vi "Farming Robot V4.vi"() -> ()   [LabVIEW 2021]
uses:
  <vilib>/myRIO/Instrument Drivers/Onboard IO/DIO/typedefs/DIO Reference.ctl
  <vilib>/myRIO/Common/Instrument Driver Framework/Utilities/typedefs/myRIO Generic Hardware Reference.ctl
  <vilib>/myRIO/Common/Instrument Driver Framework/Utilities/typedefs/Hardware Version Enum.ctl
  <vilib>/myRIO/Common/Instrument Driver Framework/Utilities/typedefs/myRIO v1.0 Reference.ctl
  <vilib>/myRIO/Common/Instrument Driver Framework/Utilities/typedefs/Generic FPGA Reference.ctl
  <vilib>/myRIO/Common/Instrument Driver Framework/myRIO v1.0/DIO/typedefs/DIO Channels List.ctl
  <vilib>/myRIO/Common/Instrument Driver Framework/myRIO v1.0/DIO/typedefs/DIO Channels Enum.ctl
  <vilib>/userDefined/High Color/nirio_resource_hc.ctl
  <vilib>/myRIO/Instrument Drivers/Onboard IO/PWM/typedefs/PWM Reference.ctl
  <vilib>/myRIO/Common/Instrument Driver Framework/myRIO v1.0/PWM/typedefs/PWM Channels Enum.ctl
  <vilib>/myRIO/Instrument Drivers/Onboard IO/PWM/typedefs/PWM Configuration.ctl
  <vilib>/myRIO/Instrument Drivers/Onboard Devices/Accelerometer/typedefs/Accelerometer Reference.ctl
  <vilib>/myRIO/Common/Instrument Driver Framework/myRIO v1.0/Accelerometer/typedefs/Accelerometer Channels List.ctl
  <vilib>/myRIO/Common/Instrument Driver Framework/myRIO v1.0/Accelerometer/typedefs/Accelerometer Channels Enum.ctl
  <vilib>/myRIO/Common/Instrument Driver Framework/Utilities/vis/Is FPGA Ref Available.vi
  <vilib>/myRIO/Common/Instrument Driver Framework/myRIO v1.0/DIO/vis/myRIO v1.1 Open DIO.vi
  <vilib>/myRIO/Instrument Drivers/Onboard IO/DIO/vis/Write.vi
  <vilib>/myRIO/Common/Instrument Driver Framework/myRIO v1.0/Accelerometer/vis/myRIO v1.1 Open Accelerometer.vi
  <vilib>/myRIO/Instrument Drivers/Onboard Devices/Accelerometer/vis/Read.vi
  <vilib>/myRIO/Common/Instrument Driver Framework/myRIO v1.0/PWM/vis/myRIO v1.1 Open PWM.vi
  <vilib>/myRIO/Instrument Drivers/Onboard IO/PWM/vis/Set Duty Cycle and Frequency.vi
  <vilib>/myRIO/Common/Instrument Driver Framework/Utilities/vis/Validate Channels.vi
  <vilib>/myRIO/Common/Instrument Driver Framework/myRIO v1.0/DIO/vis/myRIO v1.0 Reserve DIO.vi
  <vilib>/myRIO/Common/Instrument Driver Framework/myRIO v1.0/Accelerometer/vis/myRIO v1.0 Reserve Accelerometer.vi
  <vilib>/myRIO/Common/Instrument Driver Framework/myRIO v1.0/PWM/vis/myRIO v1.0 Reserve PWM.vi
  <vilib>/myRIO/Common/Instrument Driver Framework/myRIO v1.0/Resource Manager/vis/myRIO v1.0 Reserve Channel List.vi
  <vilib>/myRIO/Common/Instrument Driver Framework/myRIO v1.0/DIO/vis/myRIO v1.0 Build MUX Configuration DIO.vi
  <vilib>/myRIO/Common/Instrument Driver Framework/myRIO v1.0/Accelerometer/vis/myRIO v1.0 Build MUX Configuration Accelerometer.vi
  <vilib>/myRIO/Common/Instrument Driver Framework/myRIO v1.0/PWM/vis/myRIO v1.0 Build MUX Configuration PWM.vi
  <vilib>/myRIO/Common/Instrument Driver Framework/myRIO v1.0/Resource Manager/vis/myRIO v1.0 Reserve Channel.vi
  <vilib>/myRIO/Common/Instrument Driver Framework/myRIO v1.0/Resource Manager/vis/myRIO v1.0 Unreserve Channel.vi
  <vilib>/myRIO/Common/Instrument Driver Framework/myRIO v1.0/Resource Manager/vis/myRIO v1.0 Create Configuration List.vi
  <vilib>/myRIO/Common/Instrument Driver Framework/myRIO v1.0/Resource Manager/vis/myRIO v1.0 Build Mutex Name.vi
  <vilib>/Utility/VariantDataType/GetNumericInfo.vi
  <vilib>/Utility/error.llb/Error Cluster From Error Code.vi
  <vilib>/myRIO/Common/Instrument Driver Framework/myRIO v1.0/myRIO v1.1 Open.vi
  <vilib>/myRIO/Common/Instrument Driver Framework/Utilities/vis/IO Manager.vi
  <vilib>/myRIO/Common/Instrument Driver Framework/Utilities/vis/Configuration Manager.vi
  <vilib>/myRIO/Common/Instrument Driver Framework/myRIO v1.0/Resource Manager/vis/myRIO v1.0 Configure IO.vi
  <vilib>/myRIO/Common/Instrument Driver Framework/myRIO v1.0/myRIO v1.0 Close.vi
  <vilib>/myRIO/Common/Instrument Driver Framework/myRIO v1.0/DIO/vis/myRIO v1.0 Write DIO.vi
  <vilib>/myRIO/Common/Instrument Driver Framework/myRIO v1.0/PWM/vis/myRIO v1.0 Write PWM.vi
  <vilib>/myRIO/Common/Instrument Driver Framework/myRIO v1.0/Accelerometer/vis/myRIO v1.0 Get Scaling Constant Accelerometer.vi
  <vilib>/myRIO/Common/Instrument Driver Framework/myRIO v1.0/Accelerometer/vis/myRIO v1.0 Read Accelerometer.vi
  <vilib>/myRIO/Express VI/Onboard Devices/LED/LED Express VI.xnode
  <vilib>/myRIO/Instrument Drivers/Onboard IO/DIO/vis/myRIO DIO Open.xnode
  <vilib>/myRIO/Express VI/Onboard IO/DO/DO Express VI.xnode
  <vilib>/myRIO/Express VI/Onboard IO/PWM/PWM Express VI.xnode
  <vilib>/myRIO/Instrument Drivers/Onboard IO/PWM/vis/myRIO PWM Open.xnode
  <vilib>/myRIO/Express VI/Onboard Devices/Accelerometer/Accelerometer Express VI.xnode
  <vilib>/myRIO/Instrument Drivers/Onboard Devices/Accelerometer/vis/myRIO Accelerometer Open.xnode
  <vilib>/myRIO/Instrument Drivers/Onboard IO/DIO/DIO.lvlib
  <vilib>/myRIO/Instrument Drivers/Onboard IO/PWM/PWM.lvlib
  <vilib>/myRIO/Instrument Drivers/Onboard Devices/Accelerometer/Accelerometer.lvlib
  <vilib>/Analysis/NI_AALPro.lvlib
panel:
  out "States":T1(ring)
  out "pulse width 2":dbl
  out "Angle 2":dbl
  out "pulse width 1":dbl
  out "Angle 1":dbl
  in  "Start Farming":bool
  out "Watering":bool
  out "Seeding\nUp":bool
  out "Seeding\nDown":bool
  out "Switching\nMode":bool
  out "Drill Up":bool
  out "Drill Down":bool
  out "Intialize":bool
  out "Message":string
  in  "stop":bool
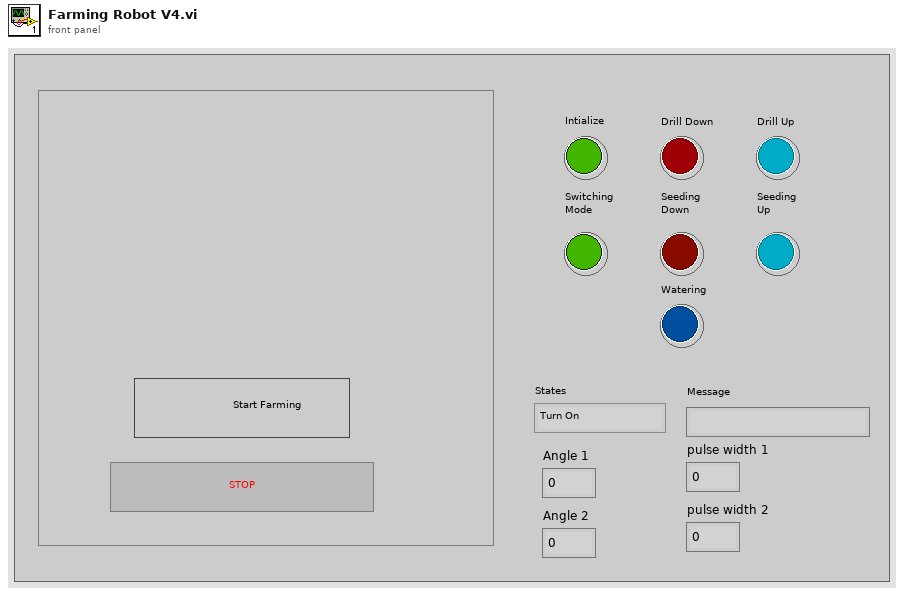
[diagram p1: front panel]
types:
  T1 = enum16{"Turn On", "IDLE", "Drive", "Down-Drilling", "Up-Drilling", "Switch-Seeding", "Down-Seeding", "Seeding", "Up-Seeding", "Switch-Watering", "Watering", "Filling", "Fell Off", "Stop"}
  T2 = typedef "DIO.lvlib/DIO Reference.ctl" = cluster{"myRIO Reference":T3, "DIO Channels List":T7}
  T3 = typedef "myRIO Generic Hardware Reference.ctl" = cluster{"myRIO Model":T4, "myRIO Hardware Reference":T5}
  T4 = typedef "Hardware Version Enum.ctl" = enum16{"Unknown", "myRIO-1900", "myRIO-1950", "roboRIO", "NI ELVIS RIO CM", "ELVIS III"}
  T5 = typedef "myRIO v1.0 Reference.ctl" = cluster{"Generic FPGA Reference":T6, "Allow multiple opens":bool}
  T6 = typedef "Generic FPGA Reference.ctl" = refnum<k20>
  T7 = typedef "DIO Channels List.ctl" = T8[]
  T8 = typedef "DIO Channels Enum.ctl" = enum16{"Not Connected", "C/DIO0", "C/DIO1", "C/DIO2", "C/DIO3", "C/DIO4", "C/DIO5", "C/DIO6", "C/DIO7", "A/DIO0", "A/DIO1", "A/DIO2", "A/DIO3", "A/DIO4", "A/DIO5", "A/DIO6", "A/DIO7", "A/DIO8", "A/DIO9", "A/DIO10", "A/DIO11", "A/DIO12", "A/DIO13", "A/DIO14", "A/DIO15", "A/DIO16", "A/DIO17", "A/DIO18", "A/DIO19", "B/DIO0", "B/DIO1", "B/DIO2", "B/DIO3", "B/DIO4", "B/DIO5", "B/DIO6", "B/DIO7", "B/DIO8", "B/DIO9", "B/DIO10", "B/DIO11", "B/DIO12", "B/DIO13", "B/DIO14", "B/DIO15", "B/DIO16", "B/DIO17", "B/DIO18", "B/DIO19", "LED0", "LED1", "LED2", "LED3", "Button0", "DIO/DIO0", "DIO/DIO1", "DIO/DIO2", "DIO/DIO3", "DIO/DIO4", "DIO/DIO5", "DIO/DIO6", "DIO/DIO7", "DIO/DIO8", "DIO/DIO9", "SPI/CS0", "SPI/CS1", "SPI/CS2", "SPI/CS3", "LED RADIO (Green)", "LED RADIO (Red)", "LED COMM (Green)", "LED COMM (Red)", "LED MODE (Green)", "LED MODE (Red)"}
  T9 = typedef "nirio_resource_hc.ctl" = tag
  T10 = typedef "Accelerometer.lvlib/Accelerometer Reference.ctl" = cluster{"myRIO Reference":T3, "Accelerometer Channels List":T11, "LSB Weight":dbl}
  T11 = typedef "Accelerometer Channels List.ctl" = T12[]
  T12 = typedef "Accelerometer Channels Enum.ctl" = enum16{"Not Connected", "X-Axis", "Y-Axis", "Z-Axis"}
  T13 = typedef "PWM.lvlib/PWM Reference.ctl" = cluster{"myRIO Reference":T3, "PWM Channels Enum":T14, "PWM Configuration":T15}
  T14 = typedef "PWM Channels Enum.ctl" = enum16{"Not Connected", "C/PWM0", "C/PWM1", "A/PWM0", "A/PWM1", "A/PWM2", "A/PWM3", "A/PWM4", "A/PWM5", "A/PWM6", "A/PWM7", "A/PWM8", "A/PWM9", "A/PWM10", "A/PWM11", "A/PWM12", "A/PWM13", "A/PWM14", "A/PWM15", "A/PWM16", "A/PWM17", "A/PWM18", "A/PWM19", "B/PWM0", "B/PWM1", "B/PWM2", "B/PWM3", "B/PWM4", "B/PWM5", "B/PWM6", "B/PWM7", "B/PWM8", "B/PWM9", "B/PWM10", "B/PWM11", "B/PWM12", "B/PWM13", "B/PWM14", "B/PWM15", "B/PWM16", "B/PWM17", "B/PWM18", "B/PWM19", "PWM/PWM0", "PWM/PWM1", "PWM/PWM2", "PWM/PWM3", "PWM/PWM4", "PWM/PWM5", "PWM/PWM6", "PWM/PWM7", "PWM/PWM8", "PWM/PWM9"}
  T15 = typedef "PWM.lvlib/PWM Configuration.ctl" = cluster{"Frequency":dbl, "Duty Cycle":dbl}
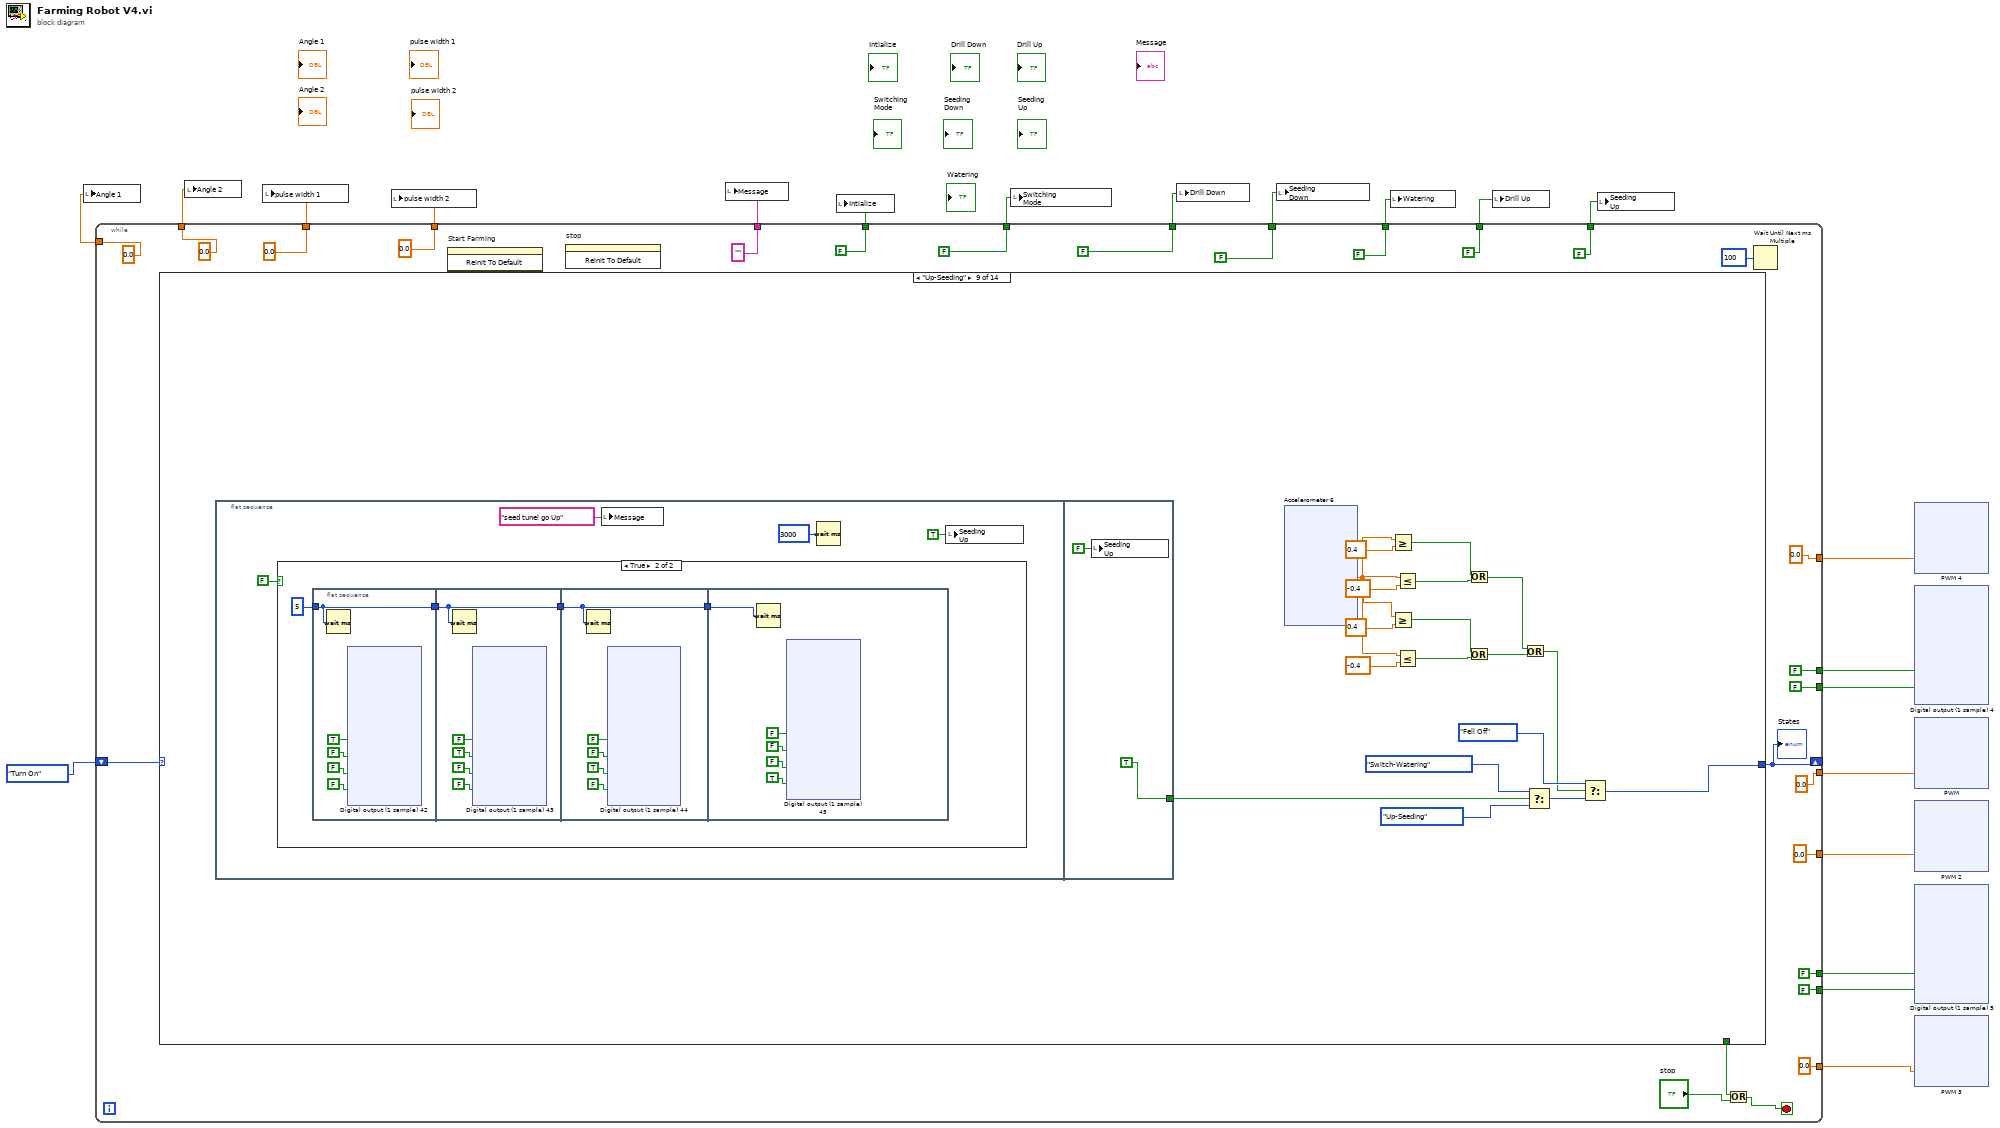
[diagram p0: block diagram]
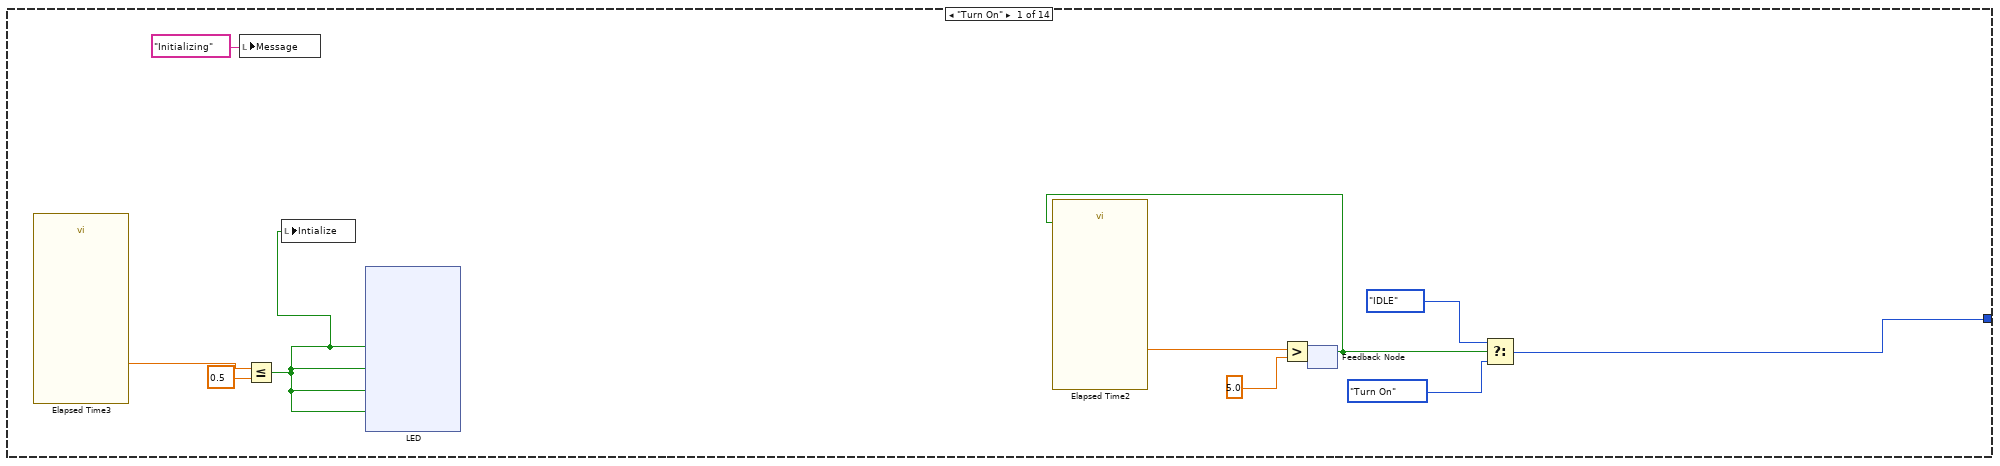
[diagram p2: hidden frame]
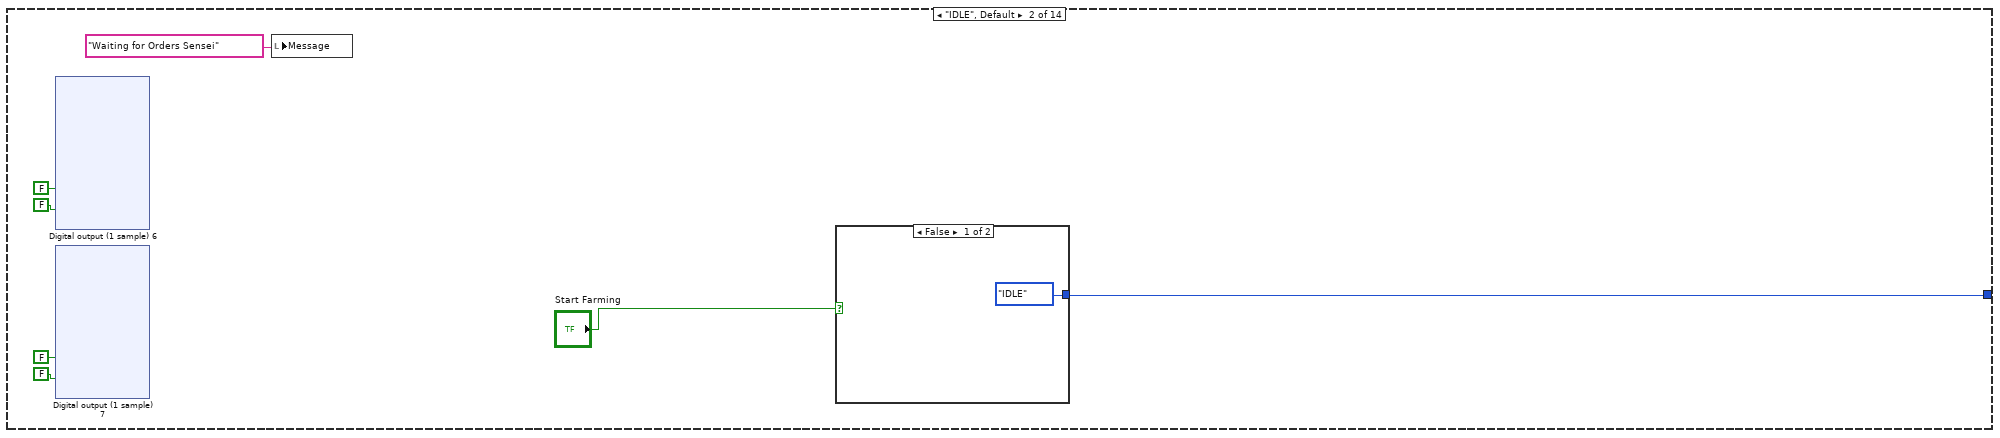
[diagram p3: hidden frame]
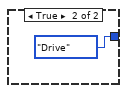
[diagram p4: hidden frame]
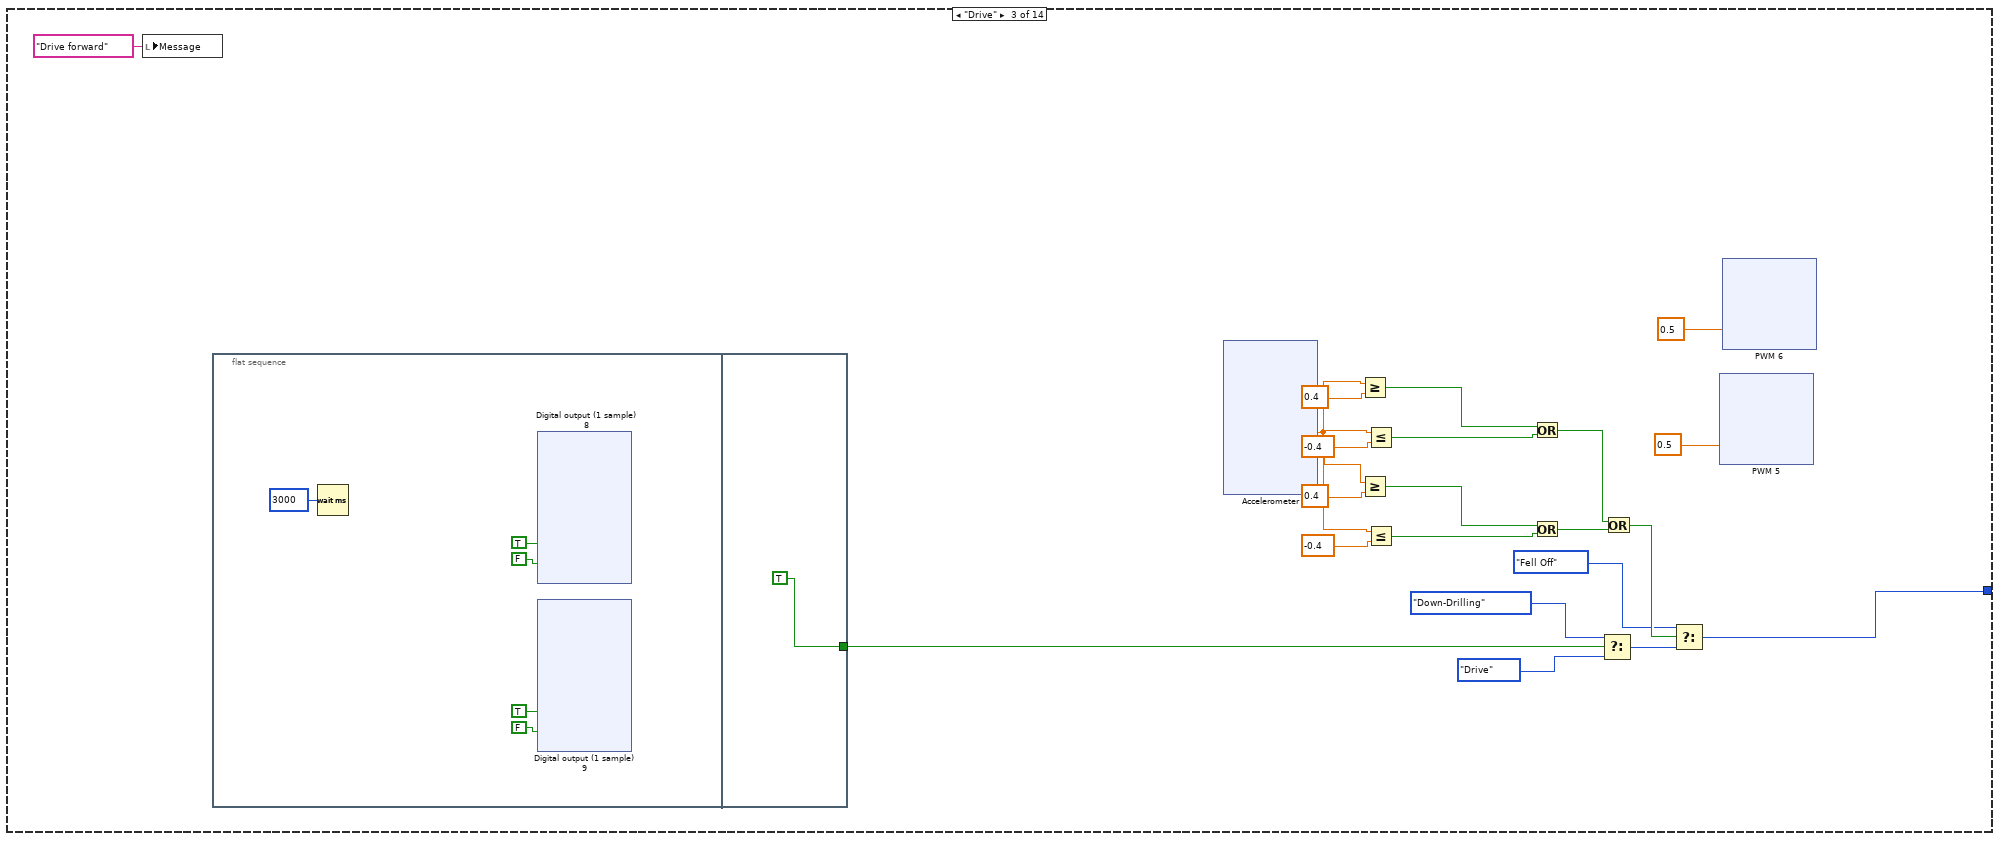
[diagram p5: hidden frame]
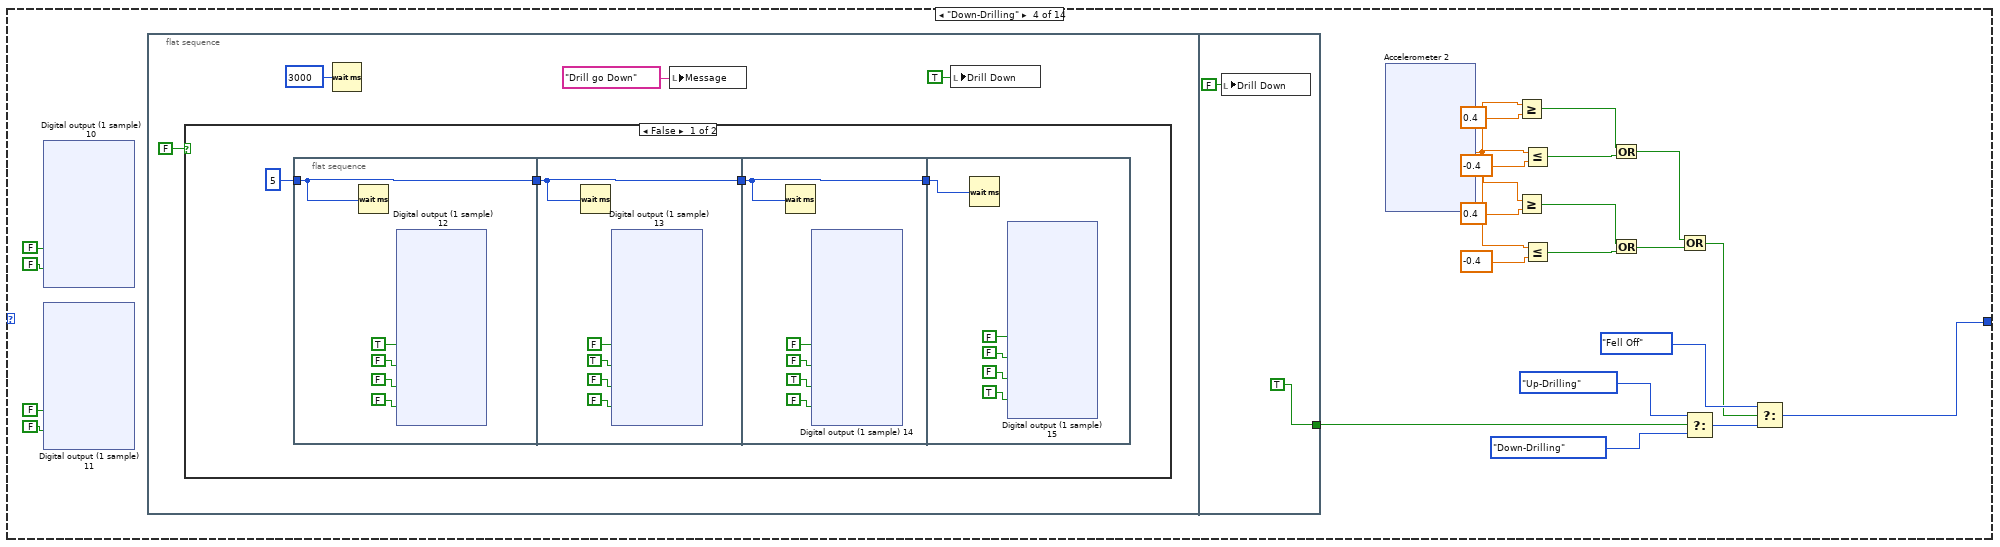
[diagram p6: hidden frame]
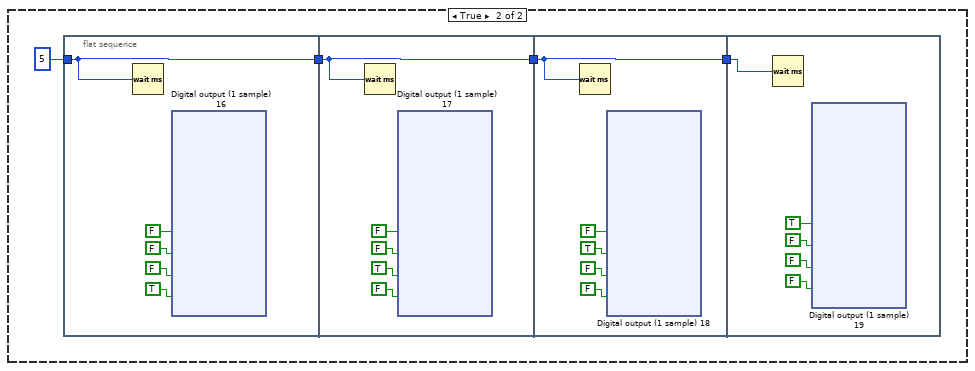
[diagram p7: hidden frame]
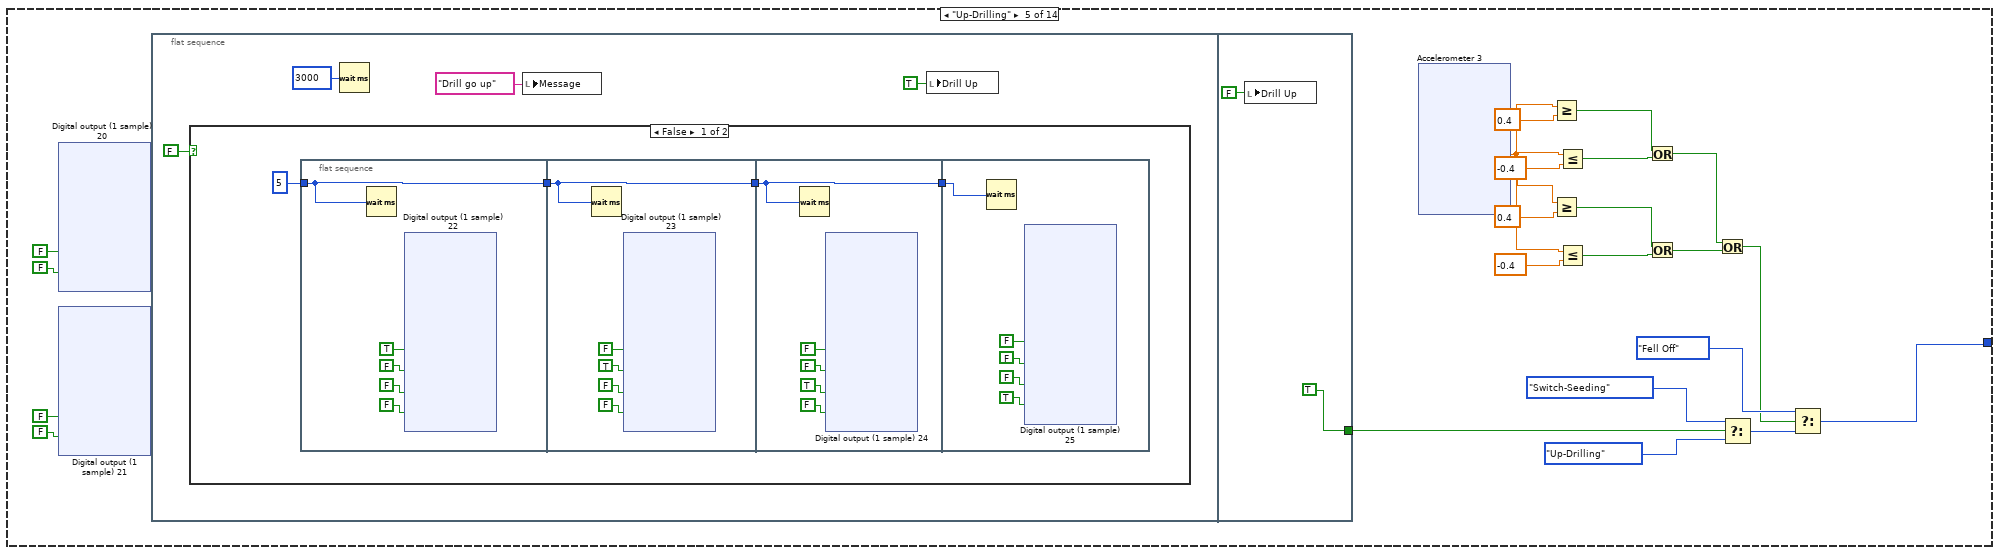
[diagram p8: hidden frame]
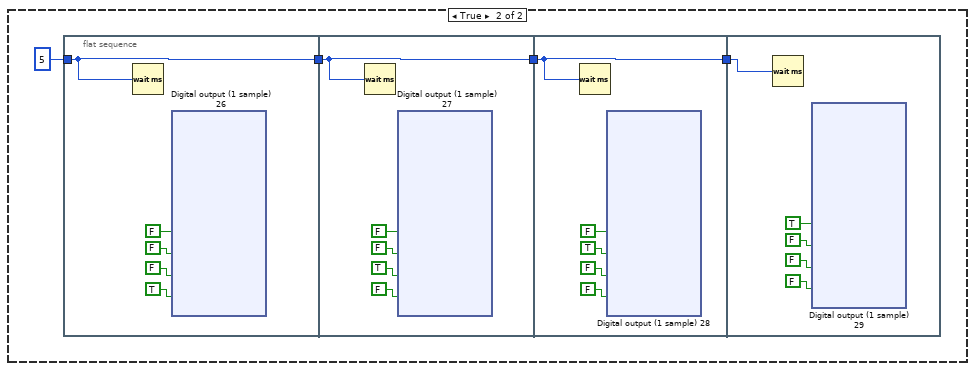
[diagram p9: hidden frame]
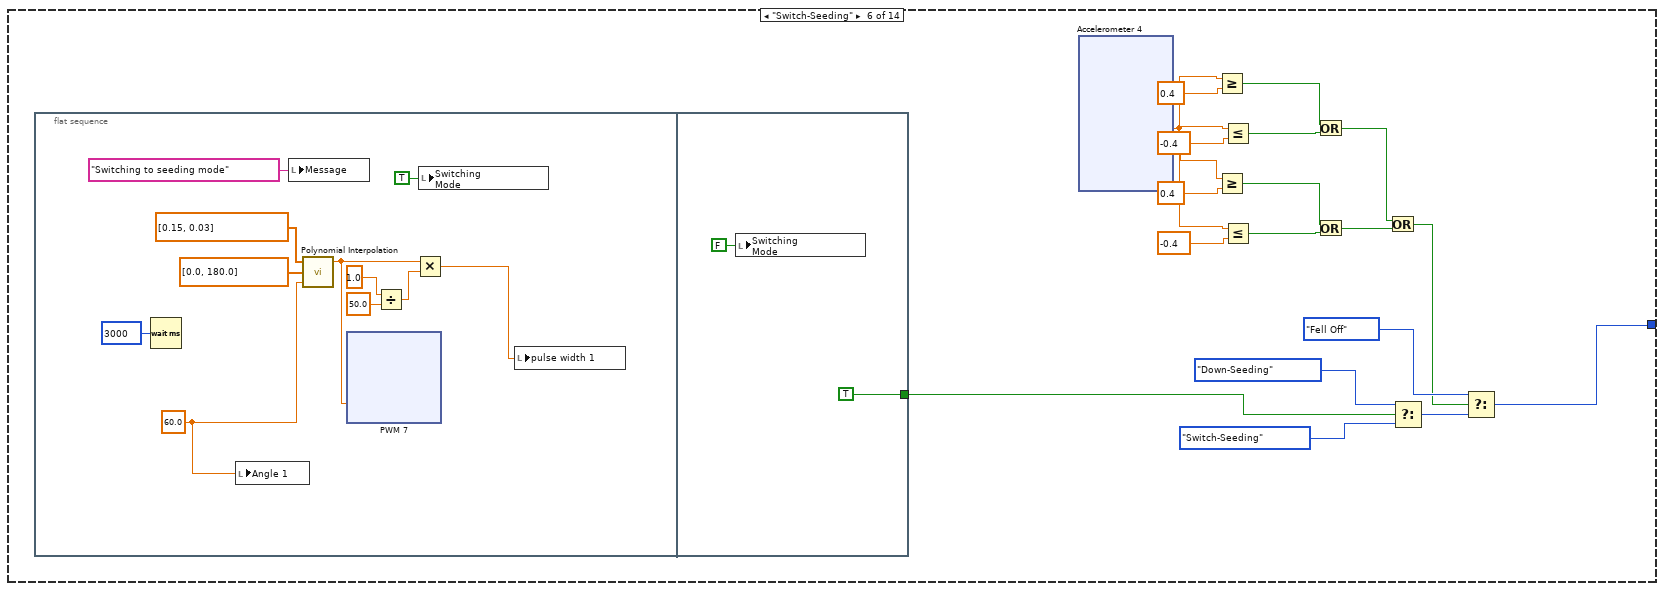
[diagram p10: hidden frame]
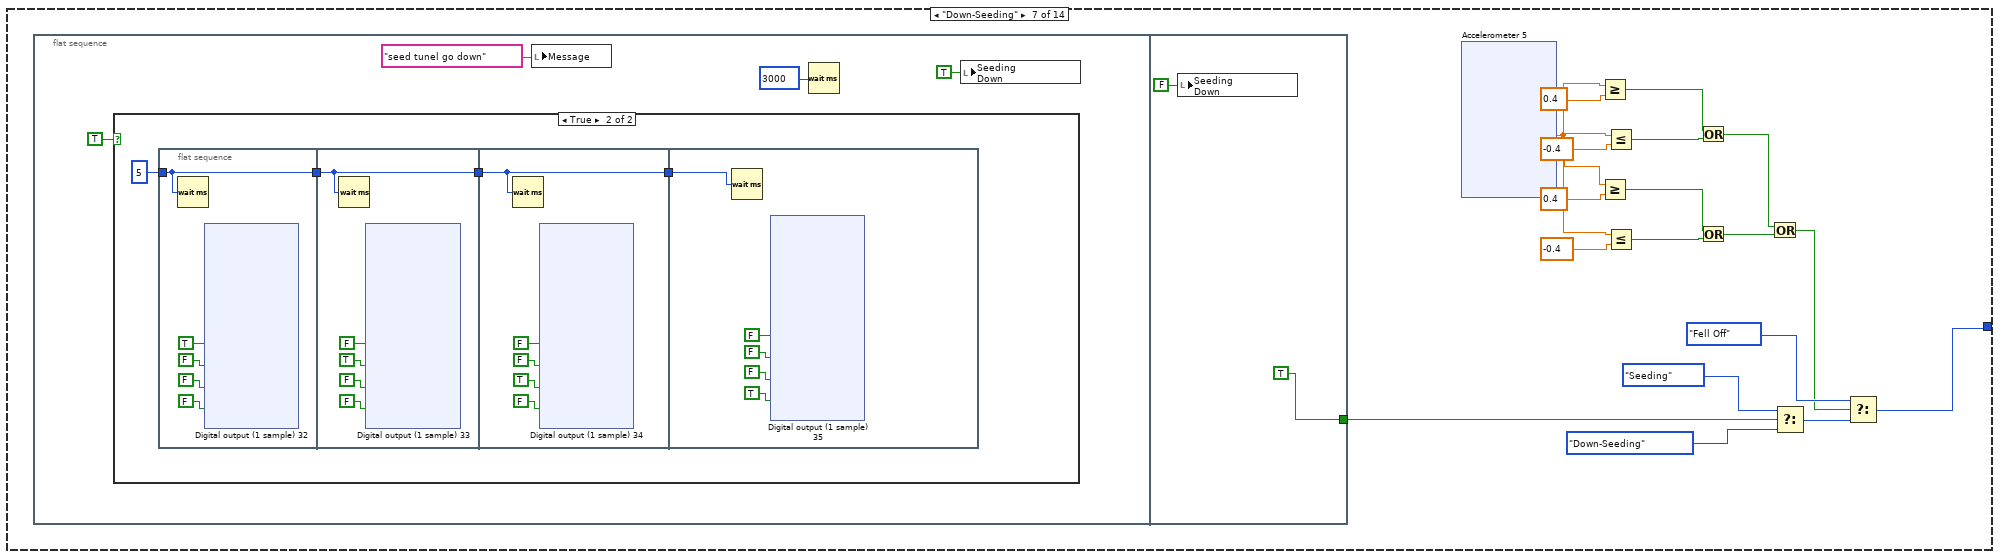
[diagram p11: hidden frame]
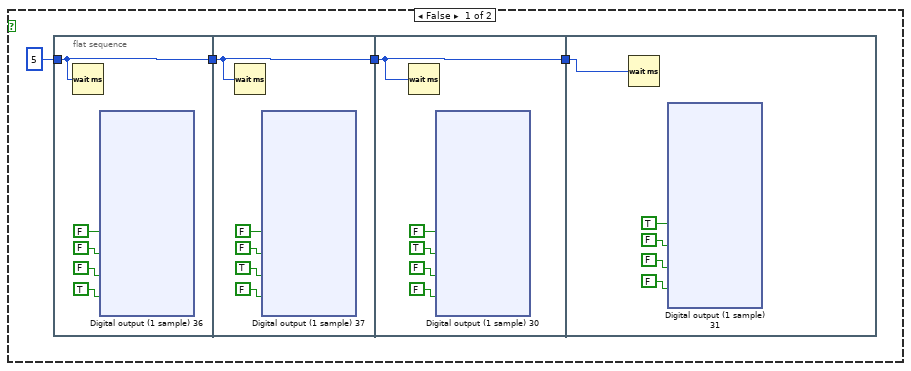
[diagram p12: hidden frame]
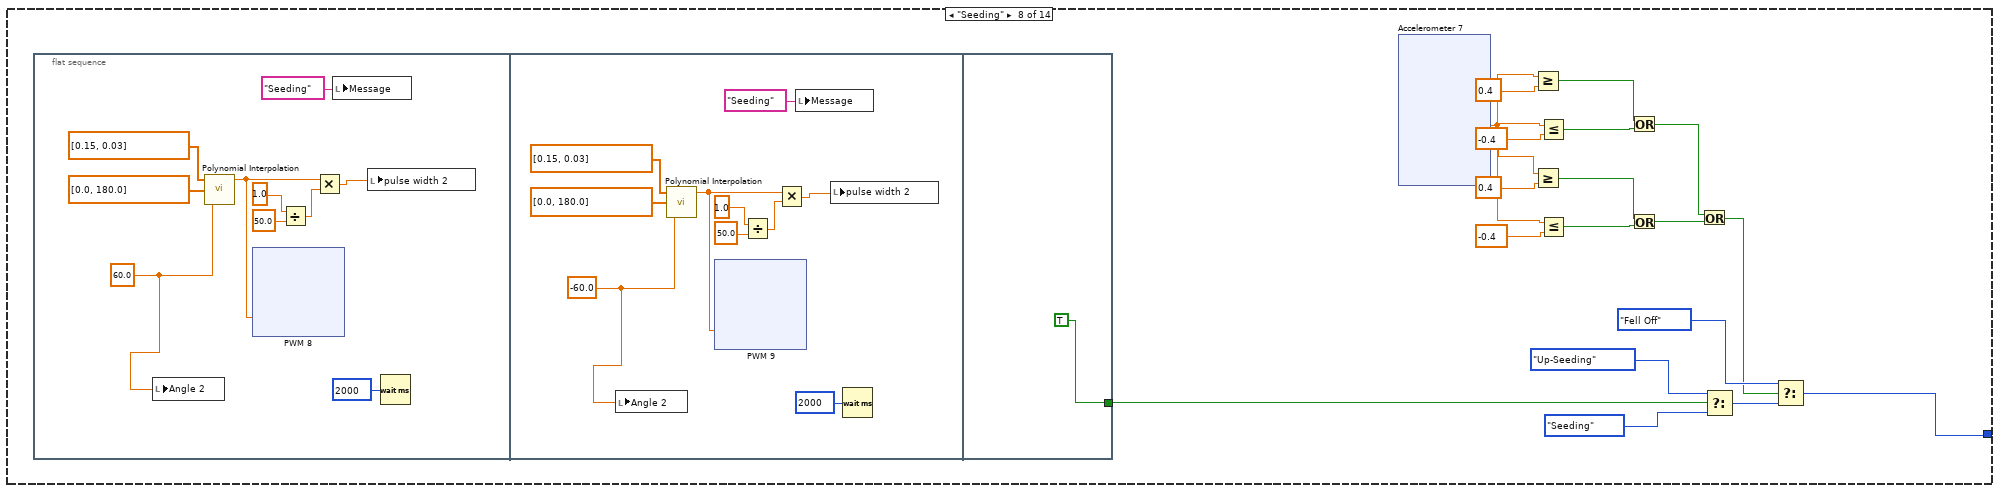
[diagram p13: hidden frame]
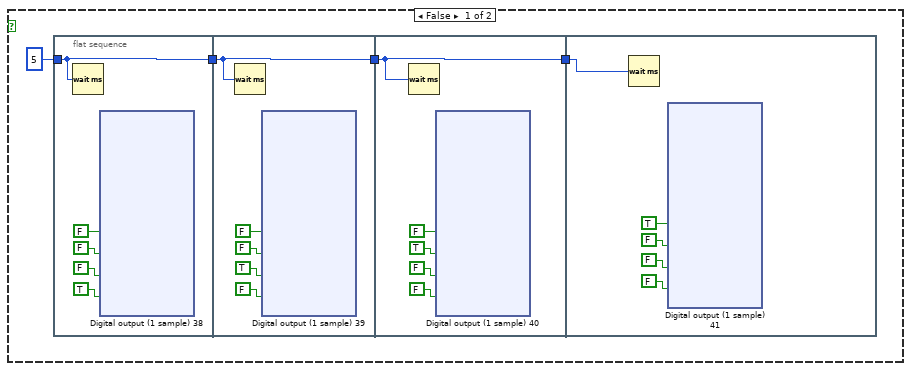
[diagram p14: hidden frame]
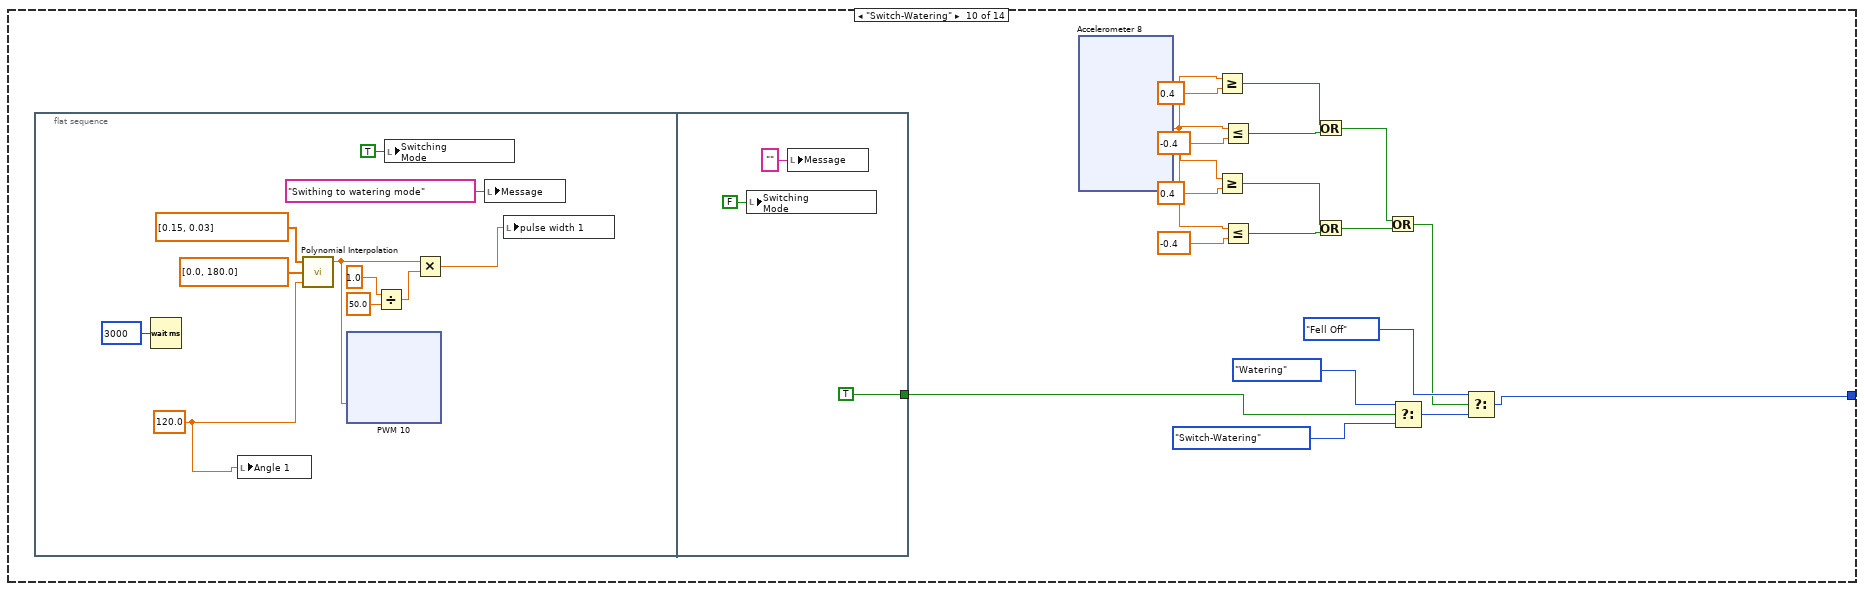
[diagram p15: hidden frame]
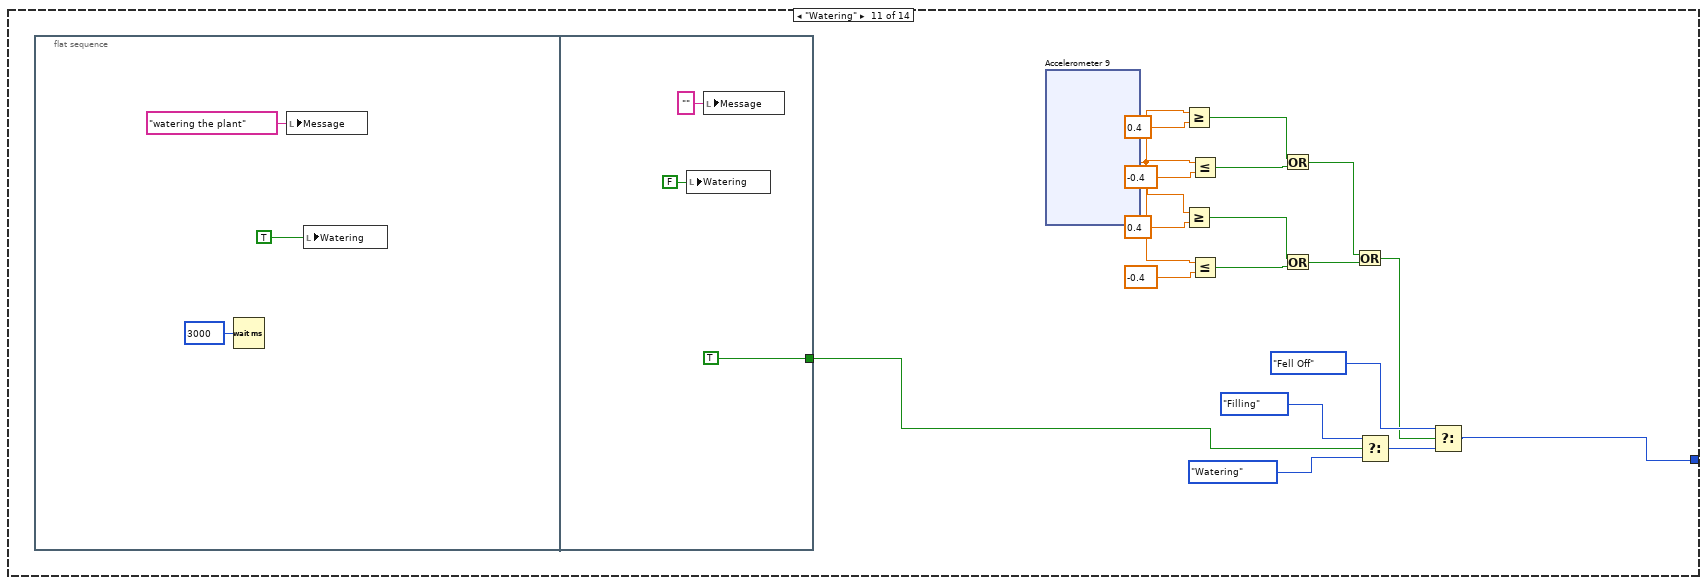
[diagram p16: hidden frame]
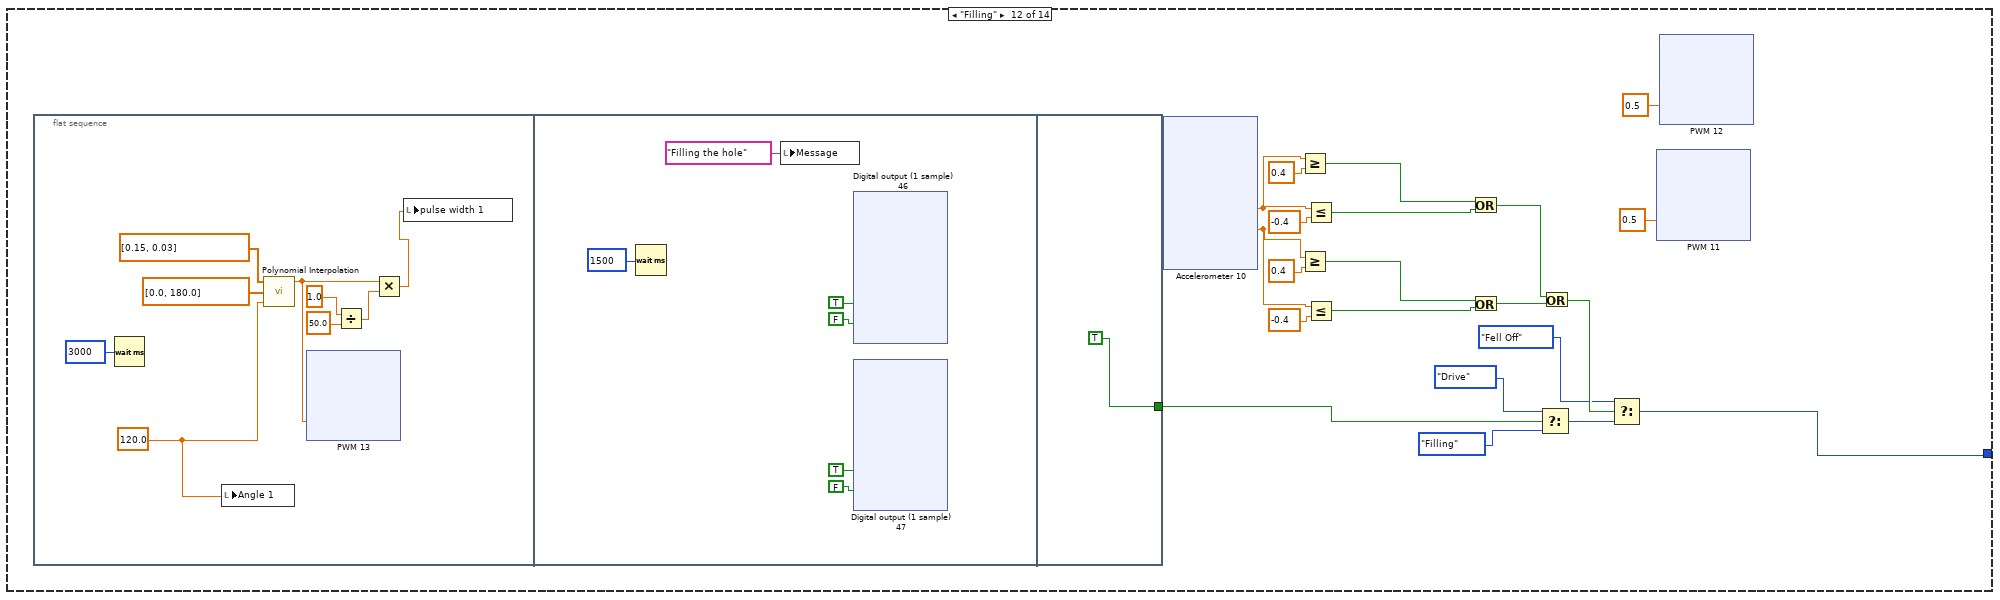
[diagram p17: hidden frame]
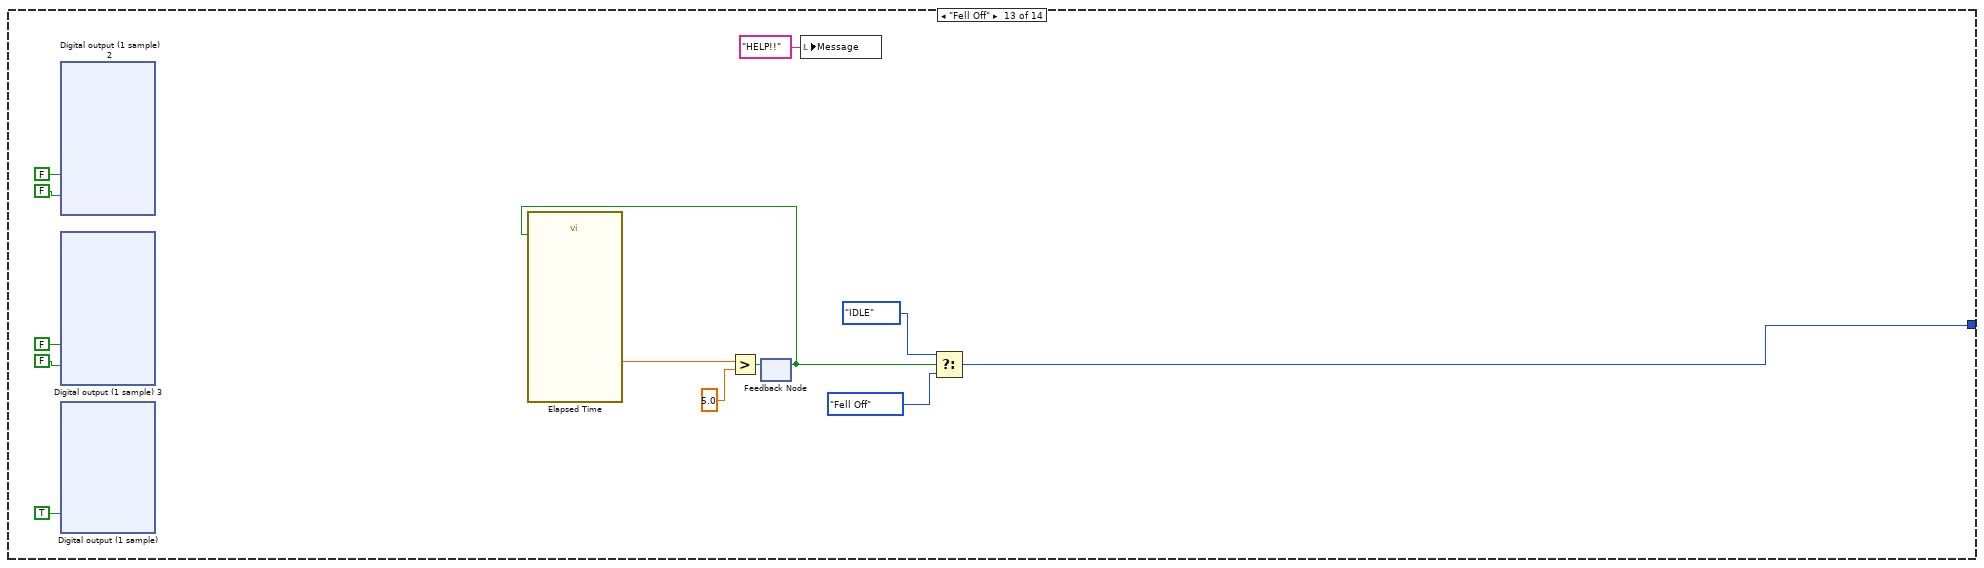
[diagram p18: hidden frame]
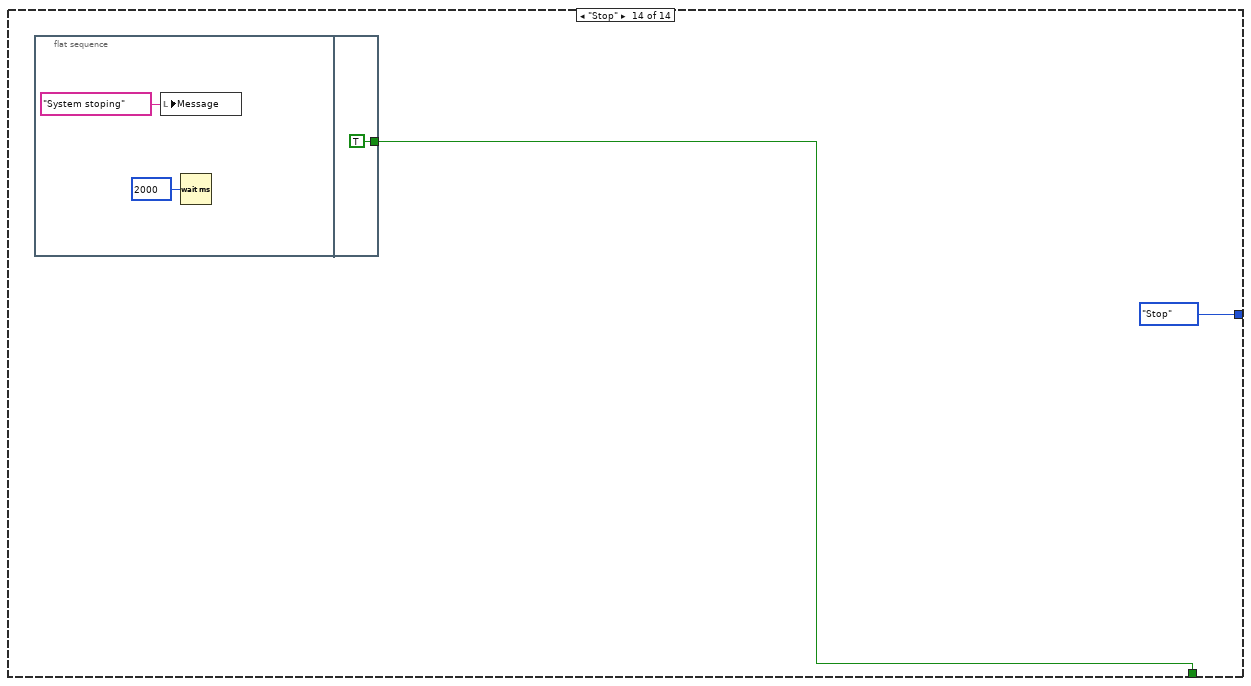
[diagram p19: hidden frame]
diagram:
  n1 = while {
    shift-right: [w42] -> _
    shift-left: T1."Turn On" ("States") -> [w45]
    tunnel: [0.0 ("Duty Cycle")] -> w20
    tunnel: [FALSE ("A/DIO1 (Pin 13)")] -> w19
    tunnel: [FALSE ("A/DIO0 (Pin 11)")] -> w18
    tunnel: [0.0 ("Duty Cycle")] -> w17
    tunnel: [0.0 ("Duty Cycle")] -> w16
    tunnel: [FALSE ("A/DIO3 (Pin 17)")] -> w15
    tunnel: [FALSE ("A/DIO2 (Pin 15)")] -> w14
    tunnel: [0.0 ("Duty Cycle")] -> w13
    tunnel: ["" ("Message")] -> w12
    tunnel: [FALSE ("Intialize")] -> w11
    tunnel: [FALSE ("Switching\nMode")] -> w10
    tunnel: [FALSE ("Drill Down")] -> w9
    tunnel: [FALSE ("Seeding\nDown")] -> w8
    tunnel: [FALSE ("Watering")] -> w7
    tunnel: [FALSE ("Drill Up")] -> w6
    tunnel: [FALSE ("Seeding\nUp")] -> w5
    tunnel: [0.0 ("pulse width 2")] -> w4
    tunnel: [0.0 ("pulse width 1")] -> w3
    tunnel: [0.0 ("Angle 2")] -> w2
    tunnel: [0.0 ("Angle 1")] -> w1
    stop <- w46 stop-if-true
    n2 = case shown="\"Up-Seeding\"" w45 {
      tunnel: [w54 w98 w183 w387 w881 w1372 w1477 w1894 w2042 w2458 w2565 w2629 w2887 T1."Stop" ("States")] -> w42
      tunnel: [_ _ _ _ _ _ _ _ _ _ _ _ _ w3002] -> w43
      frame "Turn On" {
        n3 = call "Elapsed Time3"() -> ("Elapsed Time (s)"=w52:dbl)  [unwired: 12 in, 7 out]
        n4 = local write "Message"("Initializing" ("Message")) -> ()
        n5 = Less Or Equal?(x=w52, y=0.5) -> (x <= y?=w50:bool)
        n6 = local write "Intialize"(w50) -> ()
        n7 = xnode "LED"("LED0"=w50, "LED1"=w50, "LED2"=w50, "LED3"=w50) -> ()  [unwired: 1 in, 1 out]
        n8 = feedback #1() -> (w48:bool)  [unwired: 1 in]
        n9 = call "Elapsed Time2"("Reset"=w48) -> ("Elapsed Time (s)"=w58:dbl)  [unwired: 11 in, 7 out]
        n10 = Greater?(x=w58, y=5.0) -> (0:w49:bool)
        n11 = feedback-in #1(w49) -> ()
        n12 = Select(t=T1."IDLE" ("States"), s=w48, f=T1."Turn On" ("States")) -> (s? t:f=w54:T1)
      }
      frame "IDLE", Default {
        n13 = xnode "Digital output (1 sample) 6"("A/DIO0 (Pin 11)"=FALSE, "A/DIO1 (Pin 13)"=FALSE) -> ()  [unwired: 1 in, 1 out]
        n14 = xnode "Digital output (1 sample) 7"("A/DIO2 (Pin 15)"=FALSE, "A/DIO3 (Pin 17)"=FALSE) -> ()  [unwired: 1 in, 1 out]
        n15 = local write "Message"("Waiting for Orders Sensei" ("Message")) -> ()
        n16 = case shown="False" "Start Farming" {
          tunnel: [T1."IDLE" ("States") T1."Drive" ("States")] -> w98
          frame False {
          }
          frame True {
          }
        }
      }
      frame "Drive" {
        n17 = local write "Message"("Drive forward" ("Message")) -> ()
        n18 = flat-sequence {
          tunnel: [TRUE] -> w179
          frame #0 {
            n19 = Wait (ms)(milliseconds to wait=u32 3000) -> ()  [unwired: 1 out]
            n20 = xnode "Digital output (1 sample) 8"("A/DIO2 (Pin 15)"=TRUE, "A/DIO3 (Pin 17)"=FALSE) -> ()  [unwired: 1 in, 1 out]
            n21 = xnode "Digital output (1 sample) 9"("A/DIO0 (Pin 11)"=TRUE, "A/DIO1 (Pin 13)"=FALSE) -> ()  [unwired: 1 in, 1 out]
          }
          frame #1 {
          }
        }
        n22 = xnode "Accelerometer"() -> ("X-Axis"=w197:dbl, "Y-Axis"=w186:dbl)  [unwired: 1 in, 2 out]
        n23 = Greater Or Equal?(x=w197, y=0.4) -> (x >= y?=w194:bool)
        n24 = Greater Or Equal?(x=w186, y=0.4) -> (x >= y?=w188:bool)
        n25 = Less Or Equal?(x=w197, y=-0.4) -> (x <= y?=w193:bool)
        n26 = Less Or Equal?(x=w186, y=-0.4) -> (x <= y?=w187:bool)
        n27 = Or(x=w194, y=w193) -> (x .or. y?=w192:bool)
        n28 = Or(x=w188, y=w187) -> (x .or. y?=w191:bool)
        n29 = Select(t=T1."Down-Drilling" ("States"), s=w179, f=T1."Drive" ("States")) -> (s? t:f=w184:T1)
        n30 = Or(x=w192, y=w191) -> (x .or. y?=w185:bool)
        n31 = Select(t=T1."Fell Off" ("States"), s=w185, f=w184) -> (s? t:f=w183:T1)
        n32 = xnode "PWM 5"("Duty Cycle"=0.5) -> ()  [unwired: 1 in, 1 out]
        n33 = xnode "PWM 6"("Duty Cycle"=0.5) -> ()  [unwired: 1 in, 1 out]
      }
      frame "Down-Drilling" {
        n34 = xnode "Digital output (1 sample) 10"("A/DIO0 (Pin 11)"=FALSE, "A/DIO1 (Pin 13)"=FALSE) -> ()  [unwired: 1 in, 1 out]
        n35 = xnode "Digital output (1 sample) 11"("A/DIO2 (Pin 15)"=FALSE, "A/DIO3 (Pin 17)"=FALSE) -> ()  [unwired: 1 in, 1 out]
        n36 = flat-sequence {
          tunnel: [TRUE ("s")] -> w388
          frame #0 {
            n37 = case shown="False" FALSE {
              frame False {
                n38 = flat-sequence {
                  tunnel: u32 5 ("milliseconds to wait") -> [w422]
                  tunnel: [w422] -> w417
                  tunnel: [w465] -> w416
                  tunnel: w417 -> [w465]
                  tunnel: [w508] -> w415
                  tunnel: w416 -> [w508]
                  tunnel: w415 -> [w551]
                  frame #0 {
                    n39 = Wait (ms)(milliseconds to wait=w422) -> ()  [unwired: 1 out]
                    n40 = xnode "Digital output (1 sample) 12"("B/DIO0 (Pin 11)"=TRUE, "B/DIO1 (Pin 13)"=FALSE, "B/DIO2 (Pin 15)"=FALSE, "B/DIO3 (Pin 17)"=FALSE) -> ()  [unwired: 1 in, 1 out]
                  }
                  frame #1 {
                    n41 = Wait (ms)(milliseconds to wait=w465) -> ()  [unwired: 1 out]
                    n42 = xnode "Digital output (1 sample) 13"("B/DIO0 (Pin 11)"=FALSE, "B/DIO1 (Pin 13)"=TRUE, "B/DIO2 (Pin 15)"=FALSE, "B/DIO3 (Pin 17)"=FALSE) -> ()  [unwired: 1 in, 1 out]
                  }
                  frame #2 {
                    n43 = Wait (ms)(milliseconds to wait=w508) -> ()  [unwired: 1 out]
                    n44 = xnode "Digital output (1 sample) 14"("B/DIO0 (Pin 11)"=FALSE, "B/DIO1 (Pin 13)"=FALSE, "B/DIO2 (Pin 15)"=TRUE, "B/DIO3 (Pin 17)"=FALSE) -> ()  [unwired: 1 in, 1 out]
                  }
                  frame #3 {
                    n45 = Wait (ms)(milliseconds to wait=w551) -> ()  [unwired: 1 out]
                    n46 = xnode "Digital output (1 sample) 15"("B/DIO0 (Pin 11)"=FALSE, "B/DIO1 (Pin 13)"=FALSE, "B/DIO2 (Pin 15)"=FALSE, "B/DIO3 (Pin 17)"=TRUE) -> ()  [unwired: 1 in, 1 out]
                  }
                }
              }
              frame True {
                n47 = flat-sequence {
                  tunnel: u32 5 ("milliseconds to wait") -> [w598]
                  tunnel: [w598] -> w590
                  tunnel: [w641] -> w591
                  tunnel: w590 -> [w641]
                  tunnel: [w684] -> w592
                  tunnel: w591 -> [w684]
                  tunnel: w592 -> [w727]
                  frame #0 {
                    n48 = Wait (ms)(milliseconds to wait=w598) -> ()  [unwired: 1 out]
                    n49 = xnode "Digital output (1 sample) 16"("B/DIO0 (Pin 11)"=FALSE, "B/DIO1 (Pin 13)"=FALSE, "B/DIO2 (Pin 15)"=FALSE, "B/DIO3 (Pin 17)"=TRUE) -> ()  [unwired: 1 in, 1 out]
                  }
                  frame #1 {
                    n50 = Wait (ms)(milliseconds to wait=w641) -> ()  [unwired: 1 out]
                    n51 = xnode "Digital output (1 sample) 17"("B/DIO0 (Pin 11)"=FALSE, "B/DIO1 (Pin 13)"=FALSE, "B/DIO2 (Pin 15)"=TRUE, "B/DIO3 (Pin 17)"=FALSE) -> ()  [unwired: 1 in, 1 out]
                  }
                  frame #2 {
                    n52 = Wait (ms)(milliseconds to wait=w684) -> ()  [unwired: 1 out]
                    n53 = xnode "Digital output (1 sample) 18"("B/DIO0 (Pin 11)"=FALSE, "B/DIO1 (Pin 13)"=TRUE, "B/DIO2 (Pin 15)"=FALSE, "B/DIO3 (Pin 17)"=FALSE) -> ()  [unwired: 1 in, 1 out]
                  }
                  frame #3 {
                    n54 = Wait (ms)(milliseconds to wait=w727) -> ()  [unwired: 1 out]
                    n55 = xnode "Digital output (1 sample) 19"("B/DIO0 (Pin 11)"=TRUE, "B/DIO1 (Pin 13)"=FALSE, "B/DIO2 (Pin 15)"=FALSE, "B/DIO3 (Pin 17)"=FALSE) -> ()  [unwired: 1 in, 1 out]
                  }
                }
              }
            }
            n56 = Wait (ms)(milliseconds to wait=u32 3000) -> ()  [unwired: 1 out]
            n57 = local write "Message"("Drill go Down" ("Message")) -> ()
            n58 = local write "Drill Down"(TRUE ("Drill Down")) -> ()
          }
          frame #1 {
            n59 = local write "Drill Down"(FALSE ("Drill Down")) -> ()
          }
        }
        n60 = xnode "Accelerometer 2"() -> ("X-Axis"=w405:dbl, "Y-Axis"=w394:dbl)  [unwired: 1 in, 2 out]
        n61 = Greater Or Equal?(x=w405, y=0.4) -> (x >= y?=w402:bool)
        n62 = Greater Or Equal?(x=w394, y=0.4) -> (x >= y?=w396:bool)
        n63 = Less Or Equal?(x=w405, y=-0.4) -> (x <= y?=w401:bool)
        n64 = Less Or Equal?(x=w394, y=-0.4) -> (x <= y?=w395:bool)
        n65 = Or(x=w402, y=w401) -> (x .or. y?=w400:bool)
        n66 = Or(x=w396, y=w395) -> (x .or. y?=w399:bool)
        n67 = Or(x=w400, y=w399) -> (x .or. y?=w389:bool)
        n68 = Select(t=T1."Up-Drilling" ("States"), s=w388, f=T1."Down-Drilling" ("States")) -> (s? t:f=w393:T1)
        n69 = Select(t=T1."Fell Off" ("States"), s=w389, f=w393) -> (s? t:f=w387:T1)
      }
      frame "Up-Drilling" {
        n70 = xnode "Digital output (1 sample) 20"("A/DIO0 (Pin 11)"=FALSE, "A/DIO1 (Pin 13)"=FALSE) -> ()  [unwired: 1 in, 1 out]
        n71 = xnode "Digital output (1 sample) 21"("A/DIO2 (Pin 15)"=FALSE, "A/DIO3 (Pin 17)"=FALSE) -> ()  [unwired: 1 in, 1 out]
        n72 = flat-sequence {
          tunnel: [TRUE ("s")] -> w879
          frame #0 {
            n73 = case shown="False" FALSE {
              frame False {
                n74 = flat-sequence {
                  tunnel: u32 5 ("milliseconds to wait") -> [w914]
                  tunnel: [w914] -> w909
                  tunnel: [w957] -> w908
                  tunnel: w909 -> [w957]
                  tunnel: [w1000] -> w907
                  tunnel: w908 -> [w1000]
                  tunnel: w907 -> [w1043]
                  frame #0 {
                    n75 = Wait (ms)(milliseconds to wait=w914) -> ()  [unwired: 1 out]
                    n76 = xnode "Digital output (1 sample) 22"("B/DIO0 (Pin 11)"=TRUE, "B/DIO1 (Pin 13)"=FALSE, "B/DIO2 (Pin 15)"=FALSE, "B/DIO3 (Pin 17)"=FALSE) -> ()  [unwired: 1 in, 1 out]
                  }
                  frame #1 {
                    n77 = Wait (ms)(milliseconds to wait=w957) -> ()  [unwired: 1 out]
                    n78 = xnode "Digital output (1 sample) 23"("B/DIO0 (Pin 11)"=FALSE, "B/DIO1 (Pin 13)"=TRUE, "B/DIO2 (Pin 15)"=FALSE, "B/DIO3 (Pin 17)"=FALSE) -> ()  [unwired: 1 in, 1 out]
                  }
                  frame #2 {
                    n79 = Wait (ms)(milliseconds to wait=w1000) -> ()  [unwired: 1 out]
                    n80 = xnode "Digital output (1 sample) 24"("B/DIO0 (Pin 11)"=FALSE, "B/DIO1 (Pin 13)"=FALSE, "B/DIO2 (Pin 15)"=TRUE, "B/DIO3 (Pin 17)"=FALSE) -> ()  [unwired: 1 in, 1 out]
                  }
                  frame #3 {
                    n81 = Wait (ms)(milliseconds to wait=w1043) -> ()  [unwired: 1 out]
                    n82 = xnode "Digital output (1 sample) 25"("B/DIO0 (Pin 11)"=FALSE, "B/DIO1 (Pin 13)"=FALSE, "B/DIO2 (Pin 15)"=FALSE, "B/DIO3 (Pin 17)"=TRUE) -> ()  [unwired: 1 in, 1 out]
                  }
                }
              }
              frame True {
                n83 = flat-sequence {
                  tunnel: u32 5 ("milliseconds to wait") -> [w1090]
                  tunnel: [w1090] -> w1082
                  tunnel: [w1133] -> w1083
                  tunnel: w1082 -> [w1133]
                  tunnel: [w1176] -> w1084
                  tunnel: w1083 -> [w1176]
                  tunnel: w1084 -> [w1219]
                  frame #0 {
                    n84 = Wait (ms)(milliseconds to wait=w1090) -> ()  [unwired: 1 out]
                    n85 = xnode "Digital output (1 sample) 26"("B/DIO0 (Pin 11)"=FALSE, "B/DIO1 (Pin 13)"=FALSE, "B/DIO2 (Pin 15)"=FALSE, "B/DIO3 (Pin 17)"=TRUE) -> ()  [unwired: 1 in, 1 out]
                  }
                  frame #1 {
                    n86 = Wait (ms)(milliseconds to wait=w1133) -> ()  [unwired: 1 out]
                    n87 = xnode "Digital output (1 sample) 27"("B/DIO0 (Pin 11)"=FALSE, "B/DIO1 (Pin 13)"=FALSE, "B/DIO2 (Pin 15)"=TRUE, "B/DIO3 (Pin 17)"=FALSE) -> ()  [unwired: 1 in, 1 out]
                  }
                  frame #2 {
                    n88 = Wait (ms)(milliseconds to wait=w1176) -> ()  [unwired: 1 out]
                    n89 = xnode "Digital output (1 sample) 28"("B/DIO0 (Pin 11)"=FALSE, "B/DIO1 (Pin 13)"=TRUE, "B/DIO2 (Pin 15)"=FALSE, "B/DIO3 (Pin 17)"=FALSE) -> ()  [unwired: 1 in, 1 out]
                  }
                  frame #3 {
                    n90 = Wait (ms)(milliseconds to wait=w1219) -> ()  [unwired: 1 out]
                    n91 = xnode "Digital output (1 sample) 29"("B/DIO0 (Pin 11)"=TRUE, "B/DIO1 (Pin 13)"=FALSE, "B/DIO2 (Pin 15)"=FALSE, "B/DIO3 (Pin 17)"=FALSE) -> ()  [unwired: 1 in, 1 out]
                  }
                }
              }
            }
            n92 = Wait (ms)(milliseconds to wait=u32 3000) -> ()  [unwired: 1 out]
            n93 = local write "Message"("Drill go up" ("Message")) -> ()
            n94 = local write "Drill Up"(TRUE ("Drill Up")) -> ()
          }
          frame #1 {
            n95 = local write "Drill Up"(FALSE ("Drill Up")) -> ()
          }
        }
        n96 = xnode "Accelerometer 3"() -> ("X-Axis"=w897:dbl, "Y-Axis"=w886:dbl)  [unwired: 1 in, 2 out]
        n97 = Greater Or Equal?(x=w897, y=0.4) -> (x >= y?=w894:bool)
        n98 = Greater Or Equal?(x=w886, y=0.4) -> (x >= y?=w888:bool)
        n99 = Less Or Equal?(x=w897, y=-0.4) -> (x <= y?=w893:bool)
        n100 = Less Or Equal?(x=w886, y=-0.4) -> (x <= y?=w887:bool)
        n101 = Or(x=w894, y=w893) -> (x .or. y?=w892:bool)
        n102 = Or(x=w888, y=w887) -> (x .or. y?=w891:bool)
        n103 = Or(x=w892, y=w891) -> (x .or. y?=w880:bool)
        n104 = Select(t=T1."Switch-Seeding" ("States"), s=w879, f=T1."Up-Drilling" ("States")) -> (s? t:f=w885:T1)
        n105 = Select(t=T1."Fell Off" ("States"), s=w880, f=w885) -> (s? t:f=w881:T1)
      }
      frame "Switch-Seeding" {
        n106 = flat-sequence {
          tunnel: [TRUE ("s")] -> w1371
          frame #0 {
            w1432 = 60.0 ("x value")
            n107 = Wait (ms)(milliseconds to wait=u32 3000) -> ()  [unwired: 1 out]
            n108 = local write "Angle 1"(w1432) -> ()
            n109 = local write "Message"("Switching to seeding mode" ("Message")) -> ()
            n110 = call <vilib>:"Polynomial Interpolation.vi"("x value"=w1432, "X"=dbl[] [0.0, 180.0], "Y"=dbl[] [0.15, 0.03]) -> ("interpolation value"=w1439:dbl)  [unwired: 2 out]
            n111 = xnode "PWM 7"("Duty Cycle"=w1439) -> ()  [unwired: 1 in, 1 out]
            n112 = Divide(x=1.0, y=50.0) -> (x/y=w1438:dbl)
            n113 = Multiply(x=w1439, y=w1438) -> (x*y=w1429:dbl)
            n114 = local write "Switching\nMode"(TRUE ("Switching\nMode")) -> ()
            n115 = local write "pulse width 1"(w1429) -> ()
          }
          frame #1 {
            n116 = local write "Switching\nMode"(FALSE ("Switching\nMode")) -> ()
          }
        }
        n117 = xnode "Accelerometer 4"() -> ("X-Axis"=w1389:dbl, "Y-Axis"=w1378:dbl)  [unwired: 1 in, 2 out]
        n118 = Greater Or Equal?(x=w1389, y=0.4) -> (x >= y?=w1386:bool)
        n119 = Greater Or Equal?(x=w1378, y=0.4) -> (x >= y?=w1380:bool)
        n120 = Less Or Equal?(x=w1389, y=-0.4) -> (x <= y?=w1385:bool)
        n121 = Less Or Equal?(x=w1378, y=-0.4) -> (x <= y?=w1379:bool)
        n122 = Or(x=w1386, y=w1385) -> (x .or. y?=w1384:bool)
        n123 = Or(x=w1380, y=w1379) -> (x .or. y?=w1383:bool)
        n124 = Or(x=w1384, y=w1383) -> (x .or. y?=w1373:bool)
        n125 = Select(t=T1."Down-Seeding" ("States"), s=w1371, f=T1."Switch-Seeding" ("States")) -> (s? t:f=w1377:T1)
        n126 = Select(t=T1."Fell Off" ("States"), s=w1373, f=w1377) -> (s? t:f=w1372:T1)
      }
      frame "Down-Seeding" {
        n127 = flat-sequence {
          tunnel: [TRUE ("s")] -> w1478
          frame #0 {
            n128 = case shown="True" TRUE {
              frame False {
                n129 = flat-sequence {
                  tunnel: u32 5 ("milliseconds to wait") -> [w1547]
                  tunnel: [w1547] -> w1542
                  tunnel: [w1590] -> w1541
                  tunnel: w1542 -> [w1590]
                  tunnel: [w1633] -> w1540
                  tunnel: w1541 -> [w1633]
                  tunnel: w1540 -> [w1676]
                  frame #0 {
                    n130 = Wait (ms)(milliseconds to wait=w1547) -> ()  [unwired: 1 out]
                    n131 = xnode "Digital output (1 sample) 36"("B/DIO4 (Pin 19)"=FALSE ("B/DIO0 (Pin 11)"), "B/DIO5 (Pin 21)"=FALSE ("B/DIO1 (Pin 13)"), "B/DIO6 (Pin 23)"=FALSE ("B/DIO2 (Pin 15)"), "B/DIO7 (Pin 25)"=TRUE ("B/DIO3 (Pin 17)")) -> ()  [unwired: 1 in, 1 out]
                  }
                  frame #1 {
                    n132 = Wait (ms)(milliseconds to wait=w1590) -> ()  [unwired: 1 out]
                    n133 = xnode "Digital output (1 sample) 37"("B/DIO4 (Pin 19)"=FALSE ("B/DIO0 (Pin 11)"), "B/DIO5 (Pin 21)"=FALSE ("B/DIO1 (Pin 13)"), "B/DIO6 (Pin 23)"=TRUE ("B/DIO2 (Pin 15)"), "B/DIO7 (Pin 25)"=FALSE ("B/DIO3 (Pin 17)")) -> ()  [unwired: 1 in, 1 out]
                  }
                  frame #2 {
                    n134 = Wait (ms)(milliseconds to wait=w1633) -> ()  [unwired: 1 out]
                    n135 = xnode "Digital output (1 sample) 30"("B/DIO4 (Pin 19)"=FALSE ("B/DIO0 (Pin 11)"), "B/DIO5 (Pin 21)"=TRUE ("B/DIO1 (Pin 13)"), "B/DIO6 (Pin 23)"=FALSE ("B/DIO2 (Pin 15)"), "B/DIO7 (Pin 25)"=FALSE ("B/DIO3 (Pin 17)")) -> ()  [unwired: 1 in, 1 out]
                  }
                  frame #3 {
                    n136 = Wait (ms)(milliseconds to wait=w1676) -> ()  [unwired: 1 out]
                    n137 = xnode "Digital output (1 sample) 31"("B/DIO4 (Pin 19)"=TRUE ("B/DIO0 (Pin 11)"), "B/DIO5 (Pin 21)"=FALSE ("B/DIO1 (Pin 13)"), "B/DIO6 (Pin 23)"=FALSE ("B/DIO2 (Pin 15)"), "B/DIO7 (Pin 25)"=FALSE ("B/DIO3 (Pin 17)")) -> ()  [unwired: 1 in, 1 out]
                  }
                }
              }
              frame True {
                n138 = flat-sequence {
                  tunnel: u32 5 ("milliseconds to wait") -> [w1723]
                  tunnel: [w1723] -> w1715
                  tunnel: [w1766] -> w1716
                  tunnel: w1715 -> [w1766]
                  tunnel: [w1809] -> w1717
                  tunnel: w1716 -> [w1809]
                  tunnel: w1717 -> [w1852]
                  frame #0 {
                    n139 = Wait (ms)(milliseconds to wait=w1723) -> ()  [unwired: 1 out]
                    n140 = xnode "Digital output (1 sample) 32"("B/DIO4 (Pin 19)"=TRUE ("B/DIO0 (Pin 11)"), "B/DIO5 (Pin 21)"=FALSE ("B/DIO1 (Pin 13)"), "B/DIO6 (Pin 23)"=FALSE ("B/DIO2 (Pin 15)"), "B/DIO7 (Pin 25)"=FALSE ("B/DIO3 (Pin 17)")) -> ()  [unwired: 1 in, 1 out]
                  }
                  frame #1 {
                    n141 = Wait (ms)(milliseconds to wait=w1766) -> ()  [unwired: 1 out]
                    n142 = xnode "Digital output (1 sample) 33"("B/DIO4 (Pin 19)"=FALSE ("B/DIO0 (Pin 11)"), "B/DIO5 (Pin 21)"=TRUE ("B/DIO1 (Pin 13)"), "B/DIO6 (Pin 23)"=FALSE ("B/DIO2 (Pin 15)"), "B/DIO7 (Pin 25)"=FALSE ("B/DIO3 (Pin 17)")) -> ()  [unwired: 1 in, 1 out]
                  }
                  frame #2 {
                    n143 = Wait (ms)(milliseconds to wait=w1809) -> ()  [unwired: 1 out]
                    n144 = xnode "Digital output (1 sample) 34"("B/DIO4 (Pin 19)"=FALSE ("B/DIO0 (Pin 11)"), "B/DIO5 (Pin 21)"=FALSE ("B/DIO1 (Pin 13)"), "B/DIO6 (Pin 23)"=TRUE ("B/DIO2 (Pin 15)"), "B/DIO7 (Pin 25)"=FALSE ("B/DIO3 (Pin 17)")) -> ()  [unwired: 1 in, 1 out]
                  }
                  frame #3 {
                    n145 = Wait (ms)(milliseconds to wait=w1852) -> ()  [unwired: 1 out]
                    n146 = xnode "Digital output (1 sample) 35"("B/DIO4 (Pin 19)"=FALSE ("B/DIO0 (Pin 11)"), "B/DIO5 (Pin 21)"=FALSE ("B/DIO1 (Pin 13)"), "B/DIO6 (Pin 23)"=FALSE ("B/DIO2 (Pin 15)"), "B/DIO7 (Pin 25)"=TRUE ("B/DIO3 (Pin 17)")) -> ()  [unwired: 1 in, 1 out]
                  }
                }
              }
            }
            n147 = local write "Message"("seed tunel go down" ("Message")) -> ()
            n148 = Wait (ms)(milliseconds to wait=u32 3000) -> ()  [unwired: 1 out]
            n149 = local write "Seeding\nDown"(TRUE ("Seeding\nDown")) -> ()
          }
          frame #1 {
            n150 = local write "Seeding\nDown"(FALSE ("Seeding\nDown")) -> ()
          }
        }
        n151 = xnode "Accelerometer 5"() -> ("X-Axis"=w1495:dbl, "Y-Axis"=w1484:dbl)  [unwired: 1 in, 2 out]
        n152 = Greater Or Equal?(x=w1495, y=0.4) -> (x >= y?=w1492:bool)
        n153 = Greater Or Equal?(x=w1484, y=0.4) -> (x >= y?=w1486:bool)
        n154 = Less Or Equal?(x=w1495, y=-0.4) -> (x <= y?=w1491:bool)
        n155 = Less Or Equal?(x=w1484, y=-0.4) -> (x <= y?=w1485:bool)
        n156 = Or(x=w1492, y=w1491) -> (x .or. y?=w1490:bool)
        n157 = Or(x=w1486, y=w1485) -> (x .or. y?=w1489:bool)
        n158 = Or(x=w1490, y=w1489) -> (x .or. y?=w1479:bool)
        n159 = Select(t=T1."Seeding" ("States"), s=w1478, f=T1."Down-Seeding" ("States")) -> (s? t:f=w1483:T1)
        n160 = Select(t=T1."Fell Off" ("States"), s=w1479, f=w1483) -> (s? t:f=w1477:T1)
      }
      frame "Seeding" {
        n161 = flat-sequence {
          tunnel: [TRUE ("s")] -> w1893
          frame #0 {
            w1953 = 60.0 ("x value")
            n162 = local write "Angle 2"(w1953) -> ()
            n163 = call <vilib>:"Polynomial Interpolation.vi"("x value"=w1953, "X"=dbl[] [0.0, 180.0], "Y"=dbl[] [0.15, 0.03]) -> ("interpolation value"=w1955:dbl)  [unwired: 2 out]
            n164 = xnode "PWM 8"("Duty Cycle"=w1955) -> ()  [unwired: 1 in, 1 out]
            n165 = Divide(x=1.0, y=50.0) -> (x/y=w1960:dbl)
            n166 = Multiply(x=w1955, y=w1960) -> (x*y=w1954:dbl)
            n167 = local write "Message"("Seeding" ("Message")) -> ()
            n168 = local write "pulse width 2"(w1954) -> ()
            n169 = Wait (ms)(milliseconds to wait=u32 2000) -> ()  [unwired: 1 out]
          }
          frame #1 {
            w2003 = -60.0 ("x value")
            n170 = local write "Angle 2"(w2003) -> ()
            n171 = call <vilib>:"Polynomial Interpolation.vi"("x value"=w2003, "X"=dbl[] [0.0, 180.0], "Y"=dbl[] [0.15, 0.03]) -> ("interpolation value"=w2001:dbl)  [unwired: 2 out]
            n172 = xnode "PWM 9"("Duty Cycle"=w2001) -> ()  [unwired: 1 in, 1 out]
            n173 = Divide(x=1.0, y=50.0) -> (x/y=w1996:dbl)
            n174 = Multiply(x=w2001, y=w1996) -> (x*y=w2002:dbl)
            n175 = local write "Message"("Seeding" ("Message")) -> ()
            n176 = local write "pulse width 2"(w2002) -> ()
            n177 = Wait (ms)(milliseconds to wait=u32 2000) -> ()  [unwired: 1 out]
          }
          frame #2 {
          }
        }
        n178 = xnode "Accelerometer 7"() -> ("X-Axis"=w1911:dbl, "Y-Axis"=w1900:dbl)  [unwired: 1 in, 2 out]
        n179 = Greater Or Equal?(x=w1911, y=0.4) -> (x >= y?=w1908:bool)
        n180 = Greater Or Equal?(x=w1900, y=0.4) -> (x >= y?=w1902:bool)
        n181 = Less Or Equal?(x=w1911, y=-0.4) -> (x <= y?=w1907:bool)
        n182 = Less Or Equal?(x=w1900, y=-0.4) -> (x <= y?=w1901:bool)
        n183 = Or(x=w1908, y=w1907) -> (x .or. y?=w1906:bool)
        n184 = Or(x=w1902, y=w1901) -> (x .or. y?=w1905:bool)
        n185 = Or(x=w1906, y=w1905) -> (x .or. y?=w1895:bool)
        n186 = Select(t=T1."Up-Seeding" ("States"), s=w1893, f=T1."Seeding" ("States")) -> (s? t:f=w1899:T1)
        n187 = Select(t=T1."Fell Off" ("States"), s=w1895, f=w1899) -> (s? t:f=w1894:T1)
      }
      frame "Up-Seeding" {
        n188 = flat-sequence {
          tunnel: [TRUE ("s")] -> w2043
          frame #0 {
            n189 = case shown="True" FALSE {
              frame False {
                n190 = flat-sequence {
                  tunnel: u32 5 ("milliseconds to wait") -> [w2112]
                  tunnel: [w2112] -> w2107
                  tunnel: [w2155] -> w2106
                  tunnel: w2107 -> [w2155]
                  tunnel: [w2198] -> w2105
                  tunnel: w2106 -> [w2198]
                  tunnel: w2105 -> [w2241]
                  frame #0 {
                    n191 = Wait (ms)(milliseconds to wait=w2112) -> ()  [unwired: 1 out]
                    n192 = xnode "Digital output (1 sample) 38"("B/DIO4 (Pin 19)"=FALSE ("B/DIO0 (Pin 11)"), "B/DIO5 (Pin 21)"=FALSE ("B/DIO1 (Pin 13)"), "B/DIO6 (Pin 23)"=FALSE ("B/DIO2 (Pin 15)"), "B/DIO7 (Pin 25)"=TRUE ("B/DIO3 (Pin 17)")) -> ()  [unwired: 1 in, 1 out]
                  }
                  frame #1 {
                    n193 = Wait (ms)(milliseconds to wait=w2155) -> ()  [unwired: 1 out]
                    n194 = xnode "Digital output (1 sample) 39"("B/DIO4 (Pin 19)"=FALSE ("B/DIO0 (Pin 11)"), "B/DIO5 (Pin 21)"=FALSE ("B/DIO1 (Pin 13)"), "B/DIO6 (Pin 23)"=TRUE ("B/DIO2 (Pin 15)"), "B/DIO7 (Pin 25)"=FALSE ("B/DIO3 (Pin 17)")) -> ()  [unwired: 1 in, 1 out]
                  }
                  frame #2 {
                    n195 = Wait (ms)(milliseconds to wait=w2198) -> ()  [unwired: 1 out]
                    n196 = xnode "Digital output (1 sample) 40"("B/DIO4 (Pin 19)"=FALSE ("B/DIO0 (Pin 11)"), "B/DIO5 (Pin 21)"=TRUE ("B/DIO1 (Pin 13)"), "B/DIO6 (Pin 23)"=FALSE ("B/DIO2 (Pin 15)"), "B/DIO7 (Pin 25)"=FALSE ("B/DIO3 (Pin 17)")) -> ()  [unwired: 1 in, 1 out]
                  }
                  frame #3 {
                    n197 = Wait (ms)(milliseconds to wait=w2241) -> ()  [unwired: 1 out]
                    n198 = xnode "Digital output (1 sample) 41"("B/DIO4 (Pin 19)"=TRUE ("B/DIO0 (Pin 11)"), "B/DIO5 (Pin 21)"=FALSE ("B/DIO1 (Pin 13)"), "B/DIO6 (Pin 23)"=FALSE ("B/DIO2 (Pin 15)"), "B/DIO7 (Pin 25)"=FALSE ("B/DIO3 (Pin 17)")) -> ()  [unwired: 1 in, 1 out]
                  }
                }
              }
              frame True {
                n199 = flat-sequence {
                  tunnel: u32 5 ("milliseconds to wait") -> [w2288]
                  tunnel: [w2288] -> w2280
                  tunnel: [w2331] -> w2281
                  tunnel: w2280 -> [w2331]
                  tunnel: [w2374] -> w2282
                  tunnel: w2281 -> [w2374]
                  tunnel: w2282 -> [w2417]
                  frame #0 {
                    n200 = Wait (ms)(milliseconds to wait=w2288) -> ()  [unwired: 1 out]
                    n201 = xnode "Digital output (1 sample) 42"("B/DIO4 (Pin 19)"=TRUE ("B/DIO0 (Pin 11)"), "B/DIO5 (Pin 21)"=FALSE ("B/DIO1 (Pin 13)"), "B/DIO6 (Pin 23)"=FALSE ("B/DIO2 (Pin 15)"), "B/DIO7 (Pin 25)"=FALSE ("B/DIO3 (Pin 17)")) -> ()  [unwired: 1 in, 1 out]
                  }
                  frame #1 {
                    n202 = Wait (ms)(milliseconds to wait=w2331) -> ()  [unwired: 1 out]
                    n203 = xnode "Digital output (1 sample) 43"("B/DIO4 (Pin 19)"=FALSE ("B/DIO0 (Pin 11)"), "B/DIO5 (Pin 21)"=TRUE ("B/DIO1 (Pin 13)"), "B/DIO6 (Pin 23)"=FALSE ("B/DIO2 (Pin 15)"), "B/DIO7 (Pin 25)"=FALSE ("B/DIO3 (Pin 17)")) -> ()  [unwired: 1 in, 1 out]
                  }
                  frame #2 {
                    n204 = Wait (ms)(milliseconds to wait=w2374) -> ()  [unwired: 1 out]
                    n205 = xnode "Digital output (1 sample) 44"("B/DIO4 (Pin 19)"=FALSE ("B/DIO0 (Pin 11)"), "B/DIO5 (Pin 21)"=FALSE ("B/DIO1 (Pin 13)"), "B/DIO6 (Pin 23)"=TRUE ("B/DIO2 (Pin 15)"), "B/DIO7 (Pin 25)"=FALSE ("B/DIO3 (Pin 17)")) -> ()  [unwired: 1 in, 1 out]
                  }
                  frame #3 {
                    n206 = Wait (ms)(milliseconds to wait=w2417) -> ()  [unwired: 1 out]
                    n207 = xnode "Digital output (1 sample) 45"("B/DIO4 (Pin 19)"=FALSE ("B/DIO0 (Pin 11)"), "B/DIO5 (Pin 21)"=FALSE ("B/DIO1 (Pin 13)"), "B/DIO6 (Pin 23)"=FALSE ("B/DIO2 (Pin 15)"), "B/DIO7 (Pin 25)"=TRUE ("B/DIO3 (Pin 17)")) -> ()  [unwired: 1 in, 1 out]
                  }
                }
              }
            }
            n208 = local write "Message"("seed tunel go Up" ("Message")) -> ()
            n209 = Wait (ms)(milliseconds to wait=u32 3000) -> ()  [unwired: 1 out]
            n210 = local write "Seeding\nUp"(TRUE ("Seeding\nUp")) -> ()
          }
          frame #1 {
            n211 = local write "Seeding\nUp"(FALSE ("Seeding\nUp")) -> ()
          }
        }
        n212 = xnode "Accelerometer 6"() -> ("X-Axis"=w2060:dbl, "Y-Axis"=w2049:dbl)  [unwired: 1 in, 2 out]
        n213 = Greater Or Equal?(x=w2060, y=0.4) -> (x >= y?=w2057:bool)
        n214 = Greater Or Equal?(x=w2049, y=0.4) -> (x >= y?=w2051:bool)
        n215 = Less Or Equal?(x=w2060, y=-0.4) -> (x <= y?=w2056:bool)
        n216 = Less Or Equal?(x=w2049, y=-0.4) -> (x <= y?=w2050:bool)
        n217 = Or(x=w2057, y=w2056) -> (x .or. y?=w2055:bool)
        n218 = Or(x=w2051, y=w2050) -> (x .or. y?=w2054:bool)
        n219 = Or(x=w2055, y=w2054) -> (x .or. y?=w2044:bool)
        n220 = Select(t=T1."Switch-Watering" ("States"), s=w2043, f=T1."Up-Seeding" ("States")) -> (s? t:f=w2048:T1)
        n221 = Select(t=T1."Fell Off" ("States"), s=w2044, f=w2048) -> (s? t:f=w2042:T1)
      }
      frame "Switch-Watering" {
        n222 = flat-sequence {
          tunnel: [TRUE ("s")] -> w2459
          frame #0 {
            w2519 = 120.0 ("x value")
            n223 = Wait (ms)(milliseconds to wait=u32 3000) -> ()  [unwired: 1 out]
            n224 = local write "Angle 1"(w2519) -> ()
            n225 = call <vilib>:"Polynomial Interpolation.vi"("x value"=w2519, "X"=dbl[] [0.0, 180.0], "Y"=dbl[] [0.15, 0.03]) -> ("interpolation value"=w2526:dbl)  [unwired: 2 out]
            n226 = xnode "PWM 10"("Duty Cycle"=w2526) -> ()  [unwired: 1 in, 1 out]
            n227 = Divide(x=1.0, y=50.0) -> (x/y=w2525:dbl)
            n228 = local write "Switching\nMode"(TRUE ("Switching\nMode")) -> ()
            n229 = Multiply(x=w2526, y=w2525) -> (x*y=w2518:dbl)
            n230 = local write "Message"("Swithing to watering mode" ("Message")) -> ()
            n231 = local write "pulse width 1"(w2518) -> ()
          }
          frame #1 {
            n232 = local write "Switching\nMode"(FALSE ("Switching\nMode")) -> ()
            n233 = local write "Message"("" ("Message")) -> ()
          }
        }
        n234 = xnode "Accelerometer 8"() -> ("X-Axis"=w2476:dbl, "Y-Axis"=w2465:dbl)  [unwired: 1 in, 2 out]
        n235 = Greater Or Equal?(x=w2476, y=0.4) -> (x >= y?=w2473:bool)
        n236 = Greater Or Equal?(x=w2465, y=0.4) -> (x >= y?=w2467:bool)
        n237 = Less Or Equal?(x=w2476, y=-0.4) -> (x <= y?=w2472:bool)
        n238 = Less Or Equal?(x=w2465, y=-0.4) -> (x <= y?=w2466:bool)
        n239 = Or(x=w2473, y=w2472) -> (x .or. y?=w2471:bool)
        n240 = Or(x=w2467, y=w2466) -> (x .or. y?=w2470:bool)
        n241 = Or(x=w2471, y=w2470) -> (x .or. y?=w2460:bool)
        n242 = Select(t=T1."Watering" ("States"), s=w2459, f=T1."Switch-Watering" ("States")) -> (s? t:f=w2464:T1)
        n243 = Select(t=T1."Fell Off" ("States"), s=w2460, f=w2464) -> (s? t:f=w2458:T1)
      }
      frame "Watering" {
        n244 = flat-sequence {
          tunnel: [TRUE] -> w2566
          frame #0 {
            n245 = Wait (ms)(milliseconds to wait=u32 3000) -> ()  [unwired: 1 out]
            n246 = local write "Message"("watering the plant" ("Message")) -> ()
            n247 = local write "Watering"(TRUE ("Switching\nMode")) -> ()
          }
          frame #1 {
            n248 = local write "Watering"(FALSE ("Watering")) -> ()
            n249 = local write "Message"("" ("Message")) -> ()
          }
        }
        n250 = xnode "Accelerometer 9"() -> ("X-Axis"=w2583:dbl, "Y-Axis"=w2572:dbl)  [unwired: 1 in, 2 out]
        n251 = Greater Or Equal?(x=w2583, y=0.4) -> (x >= y?=w2580:bool)
        n252 = Greater Or Equal?(x=w2572, y=0.4) -> (x >= y?=w2574:bool)
        n253 = Less Or Equal?(x=w2583, y=-0.4) -> (x <= y?=w2579:bool)
        n254 = Less Or Equal?(x=w2572, y=-0.4) -> (x <= y?=w2573:bool)
        n255 = Or(x=w2580, y=w2579) -> (x .or. y?=w2578:bool)
        n256 = Or(x=w2574, y=w2573) -> (x .or. y?=w2577:bool)
        n257 = Or(x=w2578, y=w2577) -> (x .or. y?=w2567:bool)
        n258 = Select(t=T1."Filling" ("States"), s=w2566, f=T1."Watering" ("States")) -> (s? t:f=w2571:T1)
        n259 = Select(t=T1."Fell Off" ("States"), s=w2567, f=w2571) -> (s? t:f=w2565:T1)
      }
      frame "Filling" {
        n260 = flat-sequence {
          tunnel: [TRUE] -> w2630
          frame #0 {
            w2650 = 120.0 ("x value")
            n261 = Wait (ms)(milliseconds to wait=u32 3000) -> ()  [unwired: 1 out]
            n262 = local write "Angle 1"(w2650) -> ()
            n263 = call <vilib>:"Polynomial Interpolation.vi"("x value"=w2650, "X"=dbl[] [0.0, 180.0], "Y"=dbl[] [0.15, 0.03]) -> ("interpolation value"=w2658:dbl)  [unwired: 2 out]
            n264 = xnode "PWM 13"("Duty Cycle"=w2658) -> ()  [unwired: 1 in, 1 out]
            n265 = Divide(x=1.0, y=50.0) -> (x/y=w2657:dbl)
            n266 = Multiply(x=w2658, y=w2657) -> (x*y=w2651:dbl)
            n267 = local write "pulse width 1"(w2651) -> ()
          }
          frame #1 {
            n268 = Wait (ms)(milliseconds to wait=u32 1500) -> ()  [unwired: 1 out]
            n269 = local write "Message"("Filling the hole" ("Message")) -> ()
            n270 = xnode "Digital output (1 sample) 46"("A/DIO2 (Pin 15)"=TRUE, "A/DIO3 (Pin 17)"=FALSE) -> ()  [unwired: 1 in, 1 out]
            n271 = xnode "Digital output (1 sample) 47"("A/DIO0 (Pin 11)"=TRUE, "A/DIO1 (Pin 13)"=FALSE) -> ()  [unwired: 1 in, 1 out]
          }
          frame #2 {
          }
        }
        n272 = xnode "Accelerometer 10"() -> ("X-Axis"=w2647:dbl, "Y-Axis"=w2636:dbl)  [unwired: 1 in, 2 out]
        n273 = Greater Or Equal?(x=w2647, y=0.4) -> (x >= y?=w2644:bool)
        n274 = Greater Or Equal?(x=w2636, y=0.4) -> (x >= y?=w2638:bool)
        n275 = Less Or Equal?(x=w2647, y=-0.4) -> (x <= y?=w2643:bool)
        n276 = Less Or Equal?(x=w2636, y=-0.4) -> (x <= y?=w2637:bool)
        n277 = Or(x=w2644, y=w2643) -> (x .or. y?=w2642:bool)
        n278 = Or(x=w2638, y=w2637) -> (x .or. y?=w2641:bool)
        n279 = Select(t=T1."Drive" ("States"), s=w2630, f=T1."Filling" ("States")) -> (s? t:f=w2634:T1)
        n280 = Or(x=w2642, y=w2641) -> (x .or. y?=w2635:bool)
        n281 = Select(t=T1."Fell Off" ("States"), s=w2635, f=w2634) -> (s? t:f=w2629:T1)
        n282 = xnode "PWM 11"("Duty Cycle"=0.5) -> ()  [unwired: 1 in, 1 out]
        n283 = xnode "PWM 12"("Duty Cycle"=0.5) -> ()  [unwired: 1 in, 1 out]
      }
      frame "Fell Off" {
        n284 = xnode "Digital output (1 sample) 2"("A/DIO0 (Pin 11)"=FALSE, "A/DIO1 (Pin 13)"=FALSE) -> ()  [unwired: 1 in, 1 out]
        n285 = xnode "Digital output (1 sample) 3"("A/DIO2 (Pin 15)"=FALSE, "A/DIO3 (Pin 17)"=FALSE) -> ()  [unwired: 1 in, 1 out]
        n286 = xnode "Digital output (1 sample)"("A/DIO4 (Pin 19)"=TRUE) -> ()  [unwired: 1 in, 1 out]
        n287 = feedback #2() -> (w2882:bool)  [unwired: 1 in]
        n288 = call "Elapsed Time"("Reset"=w2882) -> ("Elapsed Time (s)"=w2889:dbl)  [unwired: 11 in, 7 out]
        n289 = Greater?(x=w2889, y=5.0) -> (0:w2883:bool)
        n290 = feedback-in #2(w2883) -> ()
        n291 = local write "Message"("HELP!!" ("Message")) -> ()
        n292 = Select(t=T1."IDLE" ("States"), s=w2882, f=T1."Fell Off" ("States")) -> (s? t:f=w2887:T1)
      }
      frame "Stop" {
        n293 = flat-sequence {
          tunnel: [TRUE] -> w3002
          frame #0 {
            n294 = local write "Message"("System stoping" ("Message")) -> ()
            n295 = Wait (ms)(milliseconds to wait=u32 2000) -> ()  [unwired: 1 out]
          }
          frame #1 {
          }
        }
      }
    }
    "States" <- w42
    n296 = invoke on="Start Farming" class="Bool" method="Reinit To Default"() -> ()  [unwired: 3 in, 3 out]
    n297 = invoke on="stop" class="Bool" method="Reinit To Default"() -> ()  [unwired: 3 in, 3 out]
    n298 = Or(x=w43, y="stop") -> (x .or. y?=w46:bool)
    n299 = Wait Until Next ms Multiple(millisecond multiple=u32 100) -> ()  [unwired: 1 out]
  }
  n300 = local write "Angle 1"(w1) -> ()
  n301 = local write "Angle 2"(w2) -> ()
  n302 = local write "pulse width 1"(w3) -> ()
  n303 = local write "pulse width 2"(w4) -> ()
  n304 = local write "Message"(w12) -> ()
  n305 = local write "Intialize"(w11) -> ()
  n306 = local write "Switching\nMode"(w10) -> ()
  n307 = local write "Drill Down"(w9) -> ()
  n308 = local write "Seeding\nDown"(w8) -> ()
  n309 = local write "Watering"(w7) -> ()
  n310 = local write "Drill Up"(w6) -> ()
  n311 = local write "Seeding\nUp"(w5) -> ()
  n312 = xnode "PWM 4"("Duty Cycle"=w20) -> ()  [unwired: 1 in, 1 out]
  n313 = xnode "Digital output (1 sample) 4"("A/DIO0 (Pin 11)"=w18, "A/DIO1 (Pin 13)"=w19) -> ()  [unwired: 1 in, 1 out]
  n314 = xnode "PWM"("Duty Cycle"=w17) -> ()  [unwired: 1 in, 1 out]
  n315 = xnode "PWM 2"("Duty Cycle"=w16) -> ()  [unwired: 1 in, 1 out]
  n316 = xnode "Digital output (1 sample) 5"("A/DIO2 (Pin 15)"=w14, "A/DIO3 (Pin 17)"=w15) -> ()  [unwired: 1 in, 1 out]
  n317 = xnode "PWM 3"("Duty Cycle"=w13) -> ()  [unwired: 1 in, 1 out]
